vi "DblMonoPMDCurrentScanSM correction.vi"() -> ()   [LabVIEW 2010]
uses:
  <vilib>/DAQmx/write.llb/DAQmx Write (Analog DBL 1Chan 1Samp).vi
  <vilib>/DAQmx/read.llb/DAQmx Read (Analog 1D DBL 1Chan NSamp).vi
  <vilib>/DAQmx/read.llb/DAQmx Read (Analog 1D DBL NChan 1Samp).vi
  <vilib>/DAQmx/write.llb/DAQmx Write (Analog 2D DBL NChan NSamp).vi
  <vilib>/DAQmx/create/channels.llb/DAQmx Create Channel (AO-Voltage-Basic).vi
  <vilib>/DAQmx/create/channels.llb/DAQmx Create Channel (AI-Voltage-Basic).vi
  <vilib>/daqmx/miscellaneous.llb/DAQmx Fill In Error Info.vi
  <vilib>/DAQmx/configure/timing.llb/DAQmx Timing (Sample Clock).vi
  <vilib>/Utility/file.llb/Write To Spreadsheet File (DBL).vi
  <vilib>/Analysis/NI_AALBase.lvlib
panel:
  out "element 2":dbl=-0.008255603353784051
  out "element":dbl=0.0008638386633684422
  out "number of samples written per channel":u32=999
  out "Waveform Chart  Y":dbl[](graph)=[-0.007933120791494438, -0.007933631209985054, -0.007934141628475668, -0.007934652046966284, -0.0079351624654569, -0.007935672883947514, -0.00793618330243813, -0.007936693720928744, -0.00793720413941936, -0.007937714557909975, -0.00793822497640059, -0.007938735394891205, -0.007939245813381821, -0.007939756231872435, -0.007940266650363051, -0.007940777068853667, -0.007941287487344281, -0.007941797905834897, -0.007942308324325511, -0.007942818742816127, -0.007943329161306743, -0.007943839579797357, -0.007944349998287973, -0.007944860416778589, -0.007945370835269203, -0.007945881253759819, -0.007946391672250435, -0.007946902090741049, -0.007947412509231665, -0.00794792292772228, -0.007948433346212895, -0.00794894376470351, -0.007949454183194125, -0.00794996460168474, -0.007950475020175356, -0.00795098543866597, -0.007951495857156586, -0.007952006275647202, -0.007952516694137816, -0.007953027112628432, -0.007953537531119048, -0.007954047949609662, -0.007954558368100278, -0.007955068786590892, -0.007955579205081508, -0.007956089623572124, -0.007956600042062738, -0.007957110460553354, -0.00795762087904397, -0.007958131297534584, -0.0079586417160252, -0.007959152134515816, -0.00795966255300643, -0.007960172971497046, -0.00796068338998766, -0.007961193808478276, -0.007961704226968892, -0.007962214645459506, -0.007962725063950122, -0.007963235482440737, -0.007963745900931352, -0.007964256319421967, -0.007964766737912583, -0.007965277156403197, -0.007965787574893813, -0.007966297993384427, -0.007966808411875043, -0.00796731883036566, -0.007967829248856273, -0.00796833966734689, -0.007968850085837505, -0.00796936050432812, -0.007969870922818735, -0.007970381341309351, -0.007970891759799965, -0.007971402178290581, -0.007971912596781195, -0.007972423015271811, -0.007972933433762427, -0.007973443852253041, -0.007973954270743657, -0.007974464689234273, -0.007974975107724887, -0.007975485526215503, -0.007975995944706119, -0.007976506363196733, -0.007977016781687348, -0.007977527200177963, -0.007978037618668578, -0.007978548037159194, -0.007979058455649808, -0.007979568874140424, -0.00798007929263104, -0.007980589711121654, -0.00798110012961227, -0.007981610548102886, -0.0079821209665935, -0.007982631385084116, -0.007983141803574732, -0.007983652222065346, -0.007984162640555962, -0.007984673059046576, -0.007985183477537192, -0.007985693896027808, -0.007986204314518422, -0.007986714733009038, -0.007987225151499654, -0.007987735569990268, -0.007988245988480884, -0.0079887564069715, -0.007989266825462114, -0.00798977724395273, -0.007990287662443344, -0.00799079808093396, -0.007991308499424575, -0.00799181891791519, -0.007992329336405805, -0.007992839754896421, -0.007993350173387035, -0.007993860591877651, -0.007994371010368267, -0.007994881428858881, -0.007995391847349497, -0.007995902265840111, -0.007996412684330727, -0.007996923102821343, -0.007997433521311957, -0.007997943939802573, -0.007998454358293189, -0.007998964776783803, -0.007999475195274419, -0.007999985613765035, -0.008000496032255649, -0.008001006450746265, -0.00800151686923688, -0.008002027287727495, -0.00800253770621811, -0.008003048124708725, -0.00800355854319934, -0.008004068961689956, -0.00800457938018057, -0.008005089798671186, -0.008005600217161802, -0.008006110635652416, -0.008006621054143032, -0.008007131472633648, -0.008007641891124262, -0.008008152309614878, -0.008008662728105492, -0.008009173146596108, -0.008009683565086724, -0.008010193983577338, -0.008010704402067954, -0.00801121482055857, -0.008011725239049184, -0.0080122356575398, -0.008012746076030416, -0.00801325649452103, -0.008013766913011646, -0.00801427733150226, -0.008014787749992876, -0.008015298168483492, -0.008015808586974106, -0.008016319005464722, -0.008016829423955337, -0.008017339842445952, -0.008017850260936567, -0.008018360679427183, -0.008018871097917797, -0.008019381516408413, -0.008019891934899027, -0.008020402353389643, -0.00802091277188026, -0.008021423190370873, -0.00802193360886149, -0.008022444027352105, -0.00802295444584272, -0.008023464864333335, -0.008023975282823951, -0.008024485701314565, -0.008024996119805181, -0.008025506538295795, -0.008026016956786411, -0.008026527375277027, -0.008027037793767641, -0.008027548212258257, -0.008028058630748873, -0.008028569049239487, -0.008029079467730103, -0.008029589886220719, -0.008030100304711333, -0.008030610723201949, -0.008031121141692563, -0.008031631560183179, -0.008032141978673794, -0.008032652397164409, -0.008033162815655024, -0.00803367323414564, -0.008034183652636254, -0.00803469407112687, -0.008035204489617486, -0.0080357149081081, -0.008036225326598716, -0.008036735745089332, -0.008037246163579946, -0.008037756582070562, -0.008038267000561176, -0.008038777419051792, -0.008039287837542408, -0.008039798256033022, -0.008040308674523638, -0.008040819093014254, -0.008041329511504868, -0.008041839929995484, -0.0080423503484861, -0.008042860766976714, -0.00804337118546733, -0.008043881603957944, -0.00804439202244856, -0.008044902440939175, -0.00804541285942979, -0.008045923277920405, -0.008046433696411021, -0.008046944114901635, -0.008047454533392251, -0.008047964951882867, -0.008048475370373481, -0.008048985788864097, -0.008049496207354711, -0.008050006625845327, -0.008050517044335943, -0.008051027462826557, -0.008051537881317173, -0.008052048299807789, -0.008052558718298403, -0.008053069136789019, -0.008053579555279635, -0.008054089973770249, -0.008054600392260865, -0.00805511081075148, -0.008055621229242095, -0.00805613164773271, -0.008056642066223325, -0.00805715248471394, -0.008057662903204556, -0.00805817332169517, -0.008058683740185786, -0.008059194158676402, -0.008059704577167016, -0.008060214995657632, -0.008060725414148248, -0.008061235832638862, -0.008061746251129478, -0.008062256669620092, -0.008062767088110708, -0.008063277506601324, -0.008063787925091938, -0.008064298343582554, -0.00806480876207317, -0.008065319180563784, -0.0080658295990544, -0.008066340017545016, -0.00806685043603563, -0.008067360854526246, -0.00806787127301686, -0.008068381691507476, -0.008068892109998092, -0.008069402528488706, -0.008069912946979322, -0.008070423365469937, -0.008070933783960552, -0.008071444202451167, -0.008071954620941783, -0.008072465039432397, -0.008072975457923013, -0.008073485876413627, -0.008073996294904243, -0.00807450671339486, -0.008075017131885473, -0.00807552755037609, -0.008076037968866705, -0.00807654838735732, -0.008077058805847935, -0.008077569224338551, -0.008078079642829165, -0.008078590061319781, -0.008079100479810395, -0.008079610898301011, -0.008080121316791627, -0.008080631735282241, -0.008081142153772857, -0.008081652572263473, -0.008082162990754087, -0.008082673409244703, -0.008083183827735319, -0.008083694246225933, -0.008084204664716549, -0.008084715083207164, -0.008085225501697779, -0.008085735920188394, -0.008086246338679009, -0.008086756757169624, -0.00808726717566024, -0.008087777594150854, -0.00808828801264147, -0.008088798431132086, -0.0080893088496227, -0.008089819268113316, -0.008090329686603932, -0.008090840105094546, -0.008091350523585162, -0.008091860942075776, -0.008092371360566392, -0.008092881779057008, -0.008093392197547622, -0.008093902616038238, -0.008094413034528854, -0.008094923453019468, -0.008095433871510084, -0.0080959442900007, -0.008096454708491314, -0.00809696512698193, -0.008097475545472544, -0.00809798596396316, -0.008098496382453775, -0.00809900680094439, -0.008099517219435005, -0.008100027637925621, -0.008100538056416235, -0.008101048474906851, -0.008101558893397467, -0.008102069311888081, -0.008102579730378697, -0.008103090148869311, -0.008103600567359927, -0.008104110985850543, -0.008104621404341157, -0.008105131822831773, -0.008105642241322389, -0.008106152659813003, -0.008106663078303619, -0.008107173496794235, -0.008107683915284849, -0.008108194333775465, -0.008108704752266079, -0.008109215170756695, -0.00810972558924731, -0.008110236007737925, -0.00811074642622854, -0.008111256844719156, -0.00811176726320977, -0.008112277681700386, -0.008112788100191002, -0.008113298518681616, -0.008113808937172232, -0.008114319355662848, -0.008114829774153462, -0.008115340192644078, -0.008115850611134692, -0.008116361029625308, -0.008116871448115924, -0.008117381866606538, -0.008117892285097154, -0.00811840270358777, -0.008118913122078384, -0.008119423540569, -0.008119933959059616, -0.00812044437755023, -0.008120954796040846, -0.00812146521453146, -0.008121975633022076, -0.008122486051512692, -0.008122996470003306, -0.008123506888493922, -0.008124017306984537, -0.008124527725475152, -0.008125038143965767, -0.008125548562456383, -0.008126058980946997, -0.008126569399437613, -0.008127079817928227, -0.008127590236418843, -0.00812810065490946, -0.008128611073400073, -0.00812912149189069, -0.008129631910381305, -0.00813014232887192, -0.008130652747362535, -0.008131163165853151, -0.008131673584343765, -0.008132184002834381, -0.008132694421324995, -0.008133204839815611, -0.008133715258306227, -0.008134225676796841, -0.008134736095287457, -0.008135246513778073, -0.008135756932268687, -0.008136267350759303, -0.008136777769249919, -0.008137288187740533, -0.008137798606231149, -0.008138309024721764, -0.008138819443212379, -0.008139329861702994, -0.008139840280193609, -0.008140350698684224, -0.00814086111717484, -0.008141371535665454, -0.00814188195415607, -0.008142392372646686, -0.0081429027911373, -0.008143413209627916, -0.008143923628118532, -0.008144434046609146, -0.008144944465099762, -0.008145454883590376, -0.008145965302080992, -0.008146475720571608, -0.008146986139062222, -0.008147496557552838, -0.008148006976043454, -0.008148517394534068, -0.008149027813024684, -0.0081495382315153, -0.008150048650005914, -0.00815055906849653, -0.008151069486987144, -0.00815157990547776, -0.008152090323968375, -0.00815260074245899, -0.008153111160949605, -0.008153621579440221, -0.008154131997930835, -0.008154642416421451, -0.008155152834912067, -0.008155663253402681, -0.008156173671893297, -0.008156684090383911, -0.008157194508874527, -0.008157704927365143, -0.008158215345855757, -0.008158725764346373, -0.008159236182836989, -0.008159746601327603, -0.008160257019818219, -0.008160767438308835, -0.008161277856799449, -0.008161788275290065, -0.008162298693780679, -0.008162809112271295, -0.00816331953076191, -0.008163829949252525, -0.00816434036774314, -0.008164850786233756, -0.00816536120472437, -0.008165871623214986, -0.008166382041705602, -0.008166892460196216, -0.008167402878686832, -0.008167913297177448, -0.008168423715668062, -0.008168934134158678, -0.008169444552649292, -0.008169954971139908, -0.008170465389630524, -0.008170975808121138, -0.008171486226611754, -0.00817199664510237, -0.008172507063592984, -0.0081730174820836, -0.008173527900574216, -0.00817403831906483, -0.008174548737555446, -0.00817505915604606, -0.008175569574536676, -0.008176079993027292, -0.008176590411517906, -0.008177100830008522, -0.008177611248499137, -0.008178121666989752, -0.008178632085480367, -0.008179142503970983, -0.008179652922461597, -0.008180163340952213, -0.008180673759442827, -0.008181184177933443, -0.00818169459642406, -0.008182205014914673, -0.00818271543340529, -0.008183225851895905, -0.00818373627038652, -0.008184246688877135, -0.008184757107367751, -0.008185267525858365, -0.008185777944348981, -0.008186288362839595, -0.008186798781330211, -0.008187309199820827, -0.008187819618311441, -0.008188330036802057, -0.008188840455292673, -0.008189350873783287, -0.008189861292273903, -0.008190371710764519, -0.008190882129255133, -0.008191392547745749, -0.008191902966236363, -0.008192413384726979, -0.008192923803217594, -0.008193434221708209, -0.008193944640198824, -0.00819445505868944, -0.008194965477180054, -0.00819547589567067, -0.008195986314161286, -0.0081964967326519, -0.008197007151142516, -0.00819751756963313, -0.008198027988123746, -0.008198538406614362, -0.008199048825104976, -0.008199559243595592, -0.008200069662086208, -0.008200580080576822, -0.008201090499067438, -0.008201600917558054, -0.008202111336048668, -0.008202621754539284, -0.008203132173029898, -0.008203642591520514, -0.00820415301001113, -0.008204663428501744, -0.00820517384699236, -0.008205684265482975, -0.00820619468397359, -0.008206705102464205, -0.008207215520954821, -0.008207725939445435, -0.008208236357936051, -0.008208746776426667, -0.008209257194917281, -0.008209767613407897, -0.008210278031898511, -0.008210788450389127, -0.008211298868879743, -0.008211809287370357, -0.008212319705860973, -0.008212830124351589, -0.008213340542842203, -0.008213850961332819, -0.008214361379823435, -0.008214871798314049, -0.008215382216804665, -0.008215892635295279, -0.008216403053785895, -0.00821691347227651, -0.008217423890767125, -0.00821793430925774, -0.008218444727748356, -0.00821895514623897, -0.008219465564729586, -0.008219975983220202, -0.008220486401710816, -0.008220996820201432, -0.008221507238692046, -0.008222017657182662, -0.008222528075673278, -0.008223038494163892, -0.008223548912654508, -0.008224059331145124, -0.008224569749635738, -0.008225080168126354, -0.00822559058661697, -0.008226101005107584, -0.0082266114235982, -0.008227121842088816, -0.00822763226057943, -0.008228142679070046, -0.00822865309756066, -0.008229163516051276, -0.008229673934541892, -0.008230184353032506, -0.008230694771523122, -0.008231205190013738, -0.008231715608504352, -0.008232226026994967, -0.008232736445485583, -0.008233246863976197, -0.008233757282466813, -0.008234267700957427, -0.008234778119448043, -0.00823528853793866, -0.008235798956429273, -0.00823630937491989, -0.008236819793410505, -0.00823733021190112, -0.008237840630391735, -0.008238351048882351, -0.008238861467372965, -0.008239371885863581, -0.008239882304354195, -0.008240392722844811, -0.008240903141335427, -0.008241413559826041, -0.008241923978316657, -0.008242434396807273, -0.008242944815297887, -0.008243455233788503, -0.008243965652279119, -0.008244476070769733, -0.008244986489260349, -0.008245496907750963, -0.008246007326241579, -0.008246517744732194, -0.008247028163222809, -0.008247538581713424, -0.00824804900020404, -0.008248559418694654, -0.00824906983718527, -0.008249580255675886, -0.0082500906741665, -0.008250601092657116, -0.00825111151114773, -0.008251621929638346, -0.008252132348128962, -0.008252642766619576, -0.008253153185110192, -0.008253663603600808, -0.008254174022091422, -0.008254684440582038, -0.008255194859072654, -0.008255705277563268, -0.008256215696053884, -0.008256726114544498, -0.008257236533035114, -0.00825774695152573, -0.008258257370016344, -0.00825876778850696, -0.008259278206997575, -0.00825978862548819, -0.008260299043978805, -0.008260809462469421, -0.008261319880960035, -0.008261830299450651, -0.008262340717941265, -0.008262851136431881, -0.008263361554922497, -0.008263871973413111, -0.008264382391903727, -0.008264892810394343, -0.008265403228884957, -0.008265913647375573, -0.008266424065866189, -0.008266934484356803, -0.008267444902847419, -0.008267955321338035, -0.008268465739828649, -0.008268976158319265, -0.008269486576809879, -0.008269996995300495, -0.00827050741379111, -0.008271017832281725, -0.00827152825077234, -0.008272038669262956, -0.00827254908775357, -0.008273059506244186, -0.008273569924734802, -0.008274080343225416, -0.008274590761716032, -0.008275101180206646, -0.008275611598697262, -0.008276122017187878, -0.008276632435678492, -0.008277142854169108, -0.008277653272659724, -0.008278163691150338, -0.008278674109640954, -0.00827918452813157, -0.008279694946622184, -0.0082802053651128, -0.008280715783603416, -0.00828122620209403, -0.008281736620584646, -0.00828224703907526, -0.008282757457565876, -0.008283267876056492, -0.008283778294547106, -0.008284288713037722, -0.008284799131528338, -0.008285309550018952, -0.008285819968509568, -0.008286330387000183, -0.008286840805490798, -0.008287351223981413, -0.008287861642472028, -0.008288372060962643, -0.00828888247945326, -0.008289392897943873, -0.00828990331643449, -0.008290413734925105, -0.00829092415341572, -0.008291434571906335, -0.008291944990396951, -0.008292455408887565, -0.008292965827378181, -0.008293476245868795, -0.008293986664359411, -0.008294497082850027, -0.008295007501340641, -0.008295517919831257, -0.008296028338321873, -0.008296538756812487, -0.008297049175303103, -0.008297559593793719, -0.008298070012284333, -0.008298580430774949, -0.008299090849265563, -0.008299601267756179, -0.008300111686246794, -0.008300622104737409, -0.008301132523228024, -0.00830164294171864, -0.008302153360209254, -0.00830266377869987, -0.008303174197190486, -0.0083036846156811, -0.008304195034171716, -0.00830470545266233, -0.008305215871152946, -0.008305726289643562, -0.008306236708134176, -0.008306747126624792, -0.008307257545115408, -0.008307767963606022, -0.008308278382096638, -0.008308788800587254, -0.008309299219077868, -0.008309809637568484, -0.008310320056059098, -0.008310830474549714, -0.00831134089304033, -0.008311851311530944, -0.00831236173002156, -0.008312872148512175, -0.00831338256700279, -0.008313892985493405, -0.008314403403984021, -0.008314913822474635, -0.008315424240965251, -0.008315934659455865, -0.008316445077946481, -0.008316955496437097, -0.008317465914927711, -0.008317976333418327, -0.008318486751908943, -0.008318997170399557, -0.008319507588890173, -0.008320018007380789, -0.008320528425871403, -0.008321038844362019, -0.008321549262852633, -0.008322059681343249, -0.008322570099833865, -0.008323080518324479, -0.008323590936815095, -0.00832410135530571, -0.008324611773796325, -0.00832512219228694, -0.008325632610777556, -0.00832614302926817, -0.008326653447758786, -0.008327163866249402, -0.008327674284740016, -0.008328184703230632, -0.008328695121721246, -0.008329205540211862, -0.008329715958702478, -0.008330226377193092, -0.008330736795683708, -0.008331247214174324, -0.008331757632664938, -0.008332268051155554, -0.00833277846964617, -0.008333288888136784, -0.0083337993066274, -0.008334309725118014, -0.00833482014360863, -0.008335330562099246, -0.00833584098058986, -0.008336351399080476, -0.008336861817571092, -0.008337372236061706, -0.008337882654552322, -0.008338393073042938, -0.008338903491533552, -0.008339413910024168, -0.008339924328514783, -0.008340434747005398, -0.008340945165496013, -0.008341455583986628, -0.008341966002477243, -0.00834247642096786, -0.008342986839458473, -0.00834349725794909, -0.008344007676439705, -0.00834451809493032, -0.008345028513420935, -0.008345538931911551, -0.008346049350402165, -0.008346559768892781, -0.008347070187383395, -0.008347580605874011, -0.008348091024364627, -0.008348601442855241, -0.008349111861345857, -0.008349622279836473, -0.008350132698327087, -0.008350643116817703, -0.008351153535308319, -0.008351663953798933, -0.008352174372289549, -0.008352684790780163, -0.008353195209270779, -0.008353705627761394, -0.008354216046252009, -0.008354726464742624, -0.00835523688323324, -0.008355747301723854, -0.00835625772021447, -0.008356768138705086, -0.0083572785571957, -0.008357788975686316, -0.00835829939417693, -0.008358809812667546, -0.008359320231158162, -0.008359830649648776, -0.008360341068139392, -0.008360851486630008, -0.008361361905120622, -0.008361872323611238, -0.008362382742101854, -0.008362893160592468, -0.008363403579083084, -0.008363913997573698, -0.008364424416064314, -0.00836493483455493, -0.008365445253045544, -0.00836595567153616, -0.008366466090026775, -0.00836697650851739, -0.008367486927008005, -0.008367997345498621, -0.008368507763989235, -0.008369018182479851, -0.008369528600970465, -0.008370039019461081, -0.008370549437951697, -0.008371059856442311, -0.008371570274932927, -0.008372080693423543, -0.008372591111914157, -0.008373101530404773, -0.008373611948895389, -0.008374122367386003, -0.008374632785876619, -0.008375143204367233, -0.008375653622857849, -0.008376164041348465, -0.008376674459839079, -0.008377184878329695, -0.00837769529682031, -0.008378205715310925, -0.00837871613380154, -0.008379226552292156, -0.00837973697078277, -0.008380247389273386, -0.008380757807764002, -0.008381268226254616, -0.008381778644745232, -0.008382289063235846, -0.008382799481726462, -0.008383309900217078, -0.008383820318707692, -0.008384330737198308, -0.008384841155688924, -0.008385351574179538, -0.008385861992670154, -0.00838637241116077, -0.008386882829651384, -0.008387393248142, -0.008387903666632614, -0.00838841408512323, -0.008388924503613846, -0.00838943492210446, -0.008389945340595076, -0.008390455759085692, -0.008390966177576306, -0.008391476596066922, -0.008391987014557538, -0.008392497433048152, -0.008393007851538768, -0.008393518270029383, -0.008394028688519998, -0.008394539107010613, -0.008395049525501228, -0.008395559943991843, -0.00839607036248246, -0.008396580780973073, -0.00839709119946369, -0.008397601617954305, -0.00839811203644492, -0.008398622454935535, -0.008399132873426151, -0.008399643291916765, -0.008400153710407381, -0.008400664128897995, -0.008401174547388611, -0.008401684965879227, -0.008402195384369841, -0.008402705802860457, -0.008403216221351073, -0.008403726639841687, -0.008404237058332303, -0.008404747476822919, -0.008405257895313533, -0.008405768313804149, -0.008406278732294763, -0.008406789150785379, -0.008407299569275994, -0.008407809987766609, -0.008408320406257224, -0.00840883082474784, -0.008409341243238454, -0.00840985166172907, -0.008410362080219686, -0.0084108724987103, -0.008411382917200916, -0.00841189333569153, -0.008412403754182146, -0.008412914172672762, -0.008413424591163376, -0.008413935009653992, -0.008414445428144608, -0.008414955846635222, -0.008415466265125838, -0.008415976683616454, -0.008416487102107068, -0.008416997520597684, -0.008417507939088298, -0.008418018357578914, -0.00841852877606953, -0.008419039194560144, -0.00841954961305076, -0.008420060031541375, -0.00842057045003199, -0.008421080868522605, -0.008421591287013221, -0.008422101705503835, -0.008422612123994451, -0.008423122542485065, -0.008423632960975681, -0.008424143379466297, -0.008424653797956911, -0.008425164216447527, -0.008425674634938143, -0.008426185053428757, -0.008426695471919373, -0.008427205890409989, -0.008427716308900603, -0.008428226727391219, -0.008428737145881835, -0.008429247564372449, -0.008429757982863065, -0.008430268401353679, -0.008430778819844295, -0.00843128923833491, -0.008431799656825525, -0.00843231007531614, -0.008432820493806756, -0.00843333091229737, -0.008433841330787986, -0.0084343517492786, -0.008434862167769216, -0.008435372586259832, -0.008435883004750446, -0.008436393423241062, -0.008436903841731678, -0.008437414260222292, -0.008437924678712908, -0.008438435097203524, -0.008438945515694138, -0.008439455934184754, -0.00843996635267537, -0.008440476771165984, -0.0084409871896566, -0.008441497608147216, -0.00844200802663783, -0.008442518445128446, -0.00844302886361906]
  out "initial y":dbl=-0.007933120791494438
  out "Final Y":dbl=-0.00844302886361906
  out "Waveform Chart X":dbl[](graph)=[0.0015088037910843937, 0.0015086913782654677, 0.0015085789654465417, 0.0015084665526276157, 0.00150835413980869, 0.001508241726989764, 0.001508129314170838, 0.001508016901351912, 0.001507904488532986, 0.00150779207571406, 0.001507679662895134, 0.0015075672500762082, 0.0015074548372572823, 0.0015073424244383563, 0.0015072300116194303, 0.0015071175988005043, 0.0015070051859815783, 0.0015068927731626523, 0.0015067803603437265, 0.0015066679475248005, 0.0015065555347058745, 0.0015064431218869486, 0.0015063307090680226, 0.0015062182962490966, 0.0015061058834301706, 0.0015059934706112446, 0.0015058810577923188, 0.0015057686449733928, 0.0015056562321544668, 0.0015055438193355408, 0.0015054314065166149, 0.0015053189936976889, 0.0015052065808787629, 0.001505094168059837, 0.0015049817552409111, 0.0015048693424219851, 0.0015047569296030591, 0.0015046445167841331, 0.0015045321039652072, 0.0015044196911462812, 0.0015043072783273554, 0.0015041948655084294, 0.0015040824526895034, 0.0015039700398705774, 0.0015038576270516514, 0.0015037452142327254, 0.0015036328014137994, 0.0015035203885948737, 0.0015034079757759477, 0.0015032955629570217, 0.0015031831501380957, 0.0015030707373191697, 0.0015029583245002437, 0.0015028459116813177, 0.001502733498862392, 0.001502621086043466, 0.00150250867322454, 0.001502396260405614, 0.001502283847586688, 0.001502171434767762, 0.001502059021948836, 0.0015019466091299102, 0.0015018341963109842, 0.0015017217834920583, 0.0015016093706731323, 0.0015014969578542063, 0.0015013845450352803, 0.0015012721322163543, 0.0015011597193974285, 0.0015010473065785025, 0.0015009348937595765, 0.0015008224809406505, 0.0015007100681217246, 0.0015005976553027986, 0.0015004852424838726, 0.0015003728296649468, 0.0015002604168460208, 0.0015001480040270948, 0.0015000355912081688, 0.0014999231783892428, 0.0014998107655703169, 0.0014996983527513909, 0.0014995859399324649, 0.001499473527113539, 0.001499361114294613, 0.0014992487014756871, 0.0014991362886567611, 0.0014990238758378351, 0.0014989114630189091, 0.0014987990501999832, 0.0014986866373810574, 0.0014985742245621314, 0.0014984618117432054, 0.0014983493989242794, 0.0014982369861053534, 0.0014981245732864274, 0.0014980121604675014, 0.0014978997476485757, 0.0014977873348296497, 0.0014976749220107237, 0.0014975625091917977, 0.0014974500963728717, 0.0014973376835539457, 0.0014972252707350197, 0.001497112857916094, 0.001497000445097168, 0.001496888032278242, 0.001496775619459316, 0.00149666320664039, 0.001496550793821464, 0.001496438381002538, 0.0014963259681836122, 0.0014962135553646862, 0.0014961011425457602, 0.0014959887297268343, 0.0014958763169079083, 0.0014957639040889823, 0.0014956514912700563, 0.0014955390784511305, 0.0014954266656322045, 0.0014953142528132785, 0.0014952018399943525, 0.0014950894271754266, 0.0014949770143565006, 0.0014948646015375746, 0.0014947521887186486, 0.0014946397758997228, 0.0014945273630807968, 0.0014944149502618708, 0.0014943025374429448, 0.0014941901246240188, 0.0014940777118050929, 0.0014939652989861669, 0.001493852886167241, 0.001493740473348315, 0.0014936280605293891, 0.0014935156477104631, 0.0014934032348915371, 0.0014932908220726111, 0.0014931784092536851, 0.0014930659964347594, 0.0014929535836158334, 0.0014928411707969074, 0.0014927287579779814, 0.0014926163451590554, 0.0014925039323401294, 0.0014923915195212034, 0.0014922791067022777, 0.0014921666938833517, 0.0014920542810644257, 0.0014919418682454997, 0.0014918294554265737, 0.0014917170426076477, 0.0014916046297887217, 0.001491492216969796, 0.00149137980415087, 0.001491267391331944, 0.001491154978513018, 0.001491042565694092, 0.001490930152875166, 0.00149081774005624, 0.0014907053272373142, 0.0014905929144183882, 0.0014904805015994622, 0.0014903680887805363, 0.0014902556759616103, 0.0014901432631426843, 0.0014900308503237583, 0.0014899184375048325, 0.0014898060246859065, 0.0014896936118669805, 0.0014895811990480545, 0.0014894687862291285, 0.0014893563734102026, 0.0014892439605912766, 0.0014891315477723508, 0.0014890191349534248, 0.0014889067221344988, 0.0014887943093155728, 0.0014886818964966468, 0.0014885694836777208, 0.0014884570708587948, 0.0014883446580398689, 0.001488232245220943, 0.001488119832402017, 0.001488007419583091, 0.0014878950067641651, 0.0014877825939452391, 0.0014876701811263131, 0.0014875577683073871, 0.0014874453554884614, 0.0014873329426695354, 0.0014872205298506094, 0.0014871081170316834, 0.0014869957042127574, 0.0014868832913938314, 0.0014867708785749054, 0.0014866584657559797, 0.0014865460529370537, 0.0014864336401181277, 0.0014863212272992017, 0.0014862088144802757, 0.0014860964016613497, 0.0014859839888424237, 0.001485871576023498, 0.001485759163204572, 0.001485646750385646, 0.00148553433756672, 0.001485421924747794, 0.001485309511928868, 0.001485197099109942, 0.001485084686291016, 0.0014849722734720902, 0.0014848598606531642, 0.0014847474478342382, 0.0014846350350153123, 0.0014845226221963863, 0.0014844102093774603, 0.0014842977965585343, 0.0014841853837396085, 0.0014840729709206825, 0.0014839605581017565, 0.0014838481452828305, 0.0014837357324639045, 0.0014836233196449786, 0.0014835109068260526, 0.0014833984940071268, 0.0014832860811882008, 0.0014831736683692748, 0.0014830612555503488, 0.0014829488427314228, 0.0014828364299124968, 0.0014827240170935709, 0.001482611604274645, 0.001482499191455719, 0.001482386778636793, 0.001482274365817867, 0.0014821619529989411, 0.0014820495401800151, 0.0014819371273610891, 0.0014818247145421634, 0.0014817123017232374, 0.0014815998889043114, 0.0014814874760853854, 0.0014813750632664594, 0.0014812626504475334, 0.0014811502376286074, 0.0014810378248096816, 0.0014809254119907557, 0.0014808129991718297, 0.0014807005863529037, 0.0014805881735339777, 0.0014804757607150517, 0.0014803633478961257, 0.0014802509350772, 0.001480138522258274, 0.001480026109439348, 0.001479913696620422, 0.001479801283801496, 0.00147968887098257, 0.001479576458163644, 0.0014794640453447182, 0.0014793516325257922, 0.0014792392197068662, 0.0014791268068879402, 0.0014790143940690142, 0.0014789019812500883, 0.0014787895684311623, 0.0014786771556122363, 0.0014785647427933105, 0.0014784523299743845, 0.0014783399171554585, 0.0014782275043365325, 0.0014781150915176065, 0.0014780026786986806, 0.0014778902658797546, 0.0014777778530608288, 0.0014776654402419028, 0.0014775530274229768, 0.0014774406146040508, 0.0014773282017851248, 0.0014772157889661988, 0.0014771033761472728, 0.001476990963328347, 0.001476878550509421, 0.001476766137690495, 0.001476653724871569, 0.0014765413120526431, 0.0014764288992337171, 0.0014763164864147911, 0.0014762040735958654, 0.0014760916607769394, 0.0014759792479580134, 0.0014758668351390874, 0.0014757544223201614, 0.0014756420095012354, 0.0014755295966823094, 0.0014754171838633836, 0.0014753047710444576, 0.0014751923582255317, 0.0014750799454066057, 0.0014749675325876797, 0.0014748551197687537, 0.0014747427069498277, 0.001474630294130902, 0.001474517881311976, 0.00147440546849305, 0.001474293055674124, 0.001474180642855198, 0.001474068230036272, 0.001473955817217346, 0.0014738434043984202, 0.0014737309915794942, 0.0014736185787605682, 0.0014735061659416422, 0.0014733937531227162, 0.0014732813403037903, 0.0014731689274848643, 0.0014730565146659383, 0.0014729441018470125, 0.0014728316890280865, 0.0014727192762091605, 0.0014726068633902345, 0.0014724944505713085, 0.0014723820377523825, 0.0014722696249334566, 0.0014721572121145308, 0.0014720447992956048, 0.0014719323864766788, 0.0014718199736577528, 0.0014717075608388268, 0.0014715951480199008, 0.0014714827352009748, 0.001471370322382049, 0.001471257909563123, 0.001471145496744197, 0.001471033083925271, 0.001470920671106345, 0.0014708082582874191, 0.0014706958454684931, 0.0014705834326495673, 0.0014704710198306414, 0.0014703586070117154, 0.0014702461941927894, 0.0014701337813738634, 0.0014700213685549374, 0.0014699089557360114, 0.0014697965429170856, 0.0014696841300981596, 0.0014695717172792336, 0.0014694593044603077, 0.0014693468916413817, 0.0014692344788224557, 0.0014691220660035297, 0.001469009653184604, 0.001468897240365678, 0.001468784827546752, 0.001468672414727826, 0.0014685600019089, 0.001468447589089974, 0.001468335176271048, 0.0014682227634521222, 0.0014681103506331962, 0.0014679979378142702, 0.0014678855249953442, 0.0014677731121764182, 0.0014676606993574922, 0.0014675482865385663, 0.0014674358737196403, 0.0014673234609007145, 0.0014672110480817885, 0.0014670986352628625, 0.0014669862224439365, 0.0014668738096250105, 0.0014667613968060845, 0.0014666489839871585, 0.0014665365711682328, 0.0014664241583493068, 0.0014663117455303808, 0.0014661993327114548, 0.0014660869198925288, 0.0014659745070736028, 0.0014658620942546768, 0.001465749681435751, 0.001465637268616825, 0.001465524855797899, 0.001465412442978973, 0.001465300030160047, 0.001465187617341121, 0.0014650752045221951, 0.0014649627917032693, 0.0014648503788843434, 0.0014647379660654174, 0.0014646255532464914, 0.0014645131404275654, 0.0014644007276086394, 0.0014642883147897134, 0.0014641759019707876, 0.0014640634891518616, 0.0014639510763329356, 0.0014638386635140097, 0.0014637262506950837, 0.0014636138378761577, 0.0014635014250572317, 0.001463389012238306, 0.00146327659941938, 0.001463164186600454, 0.001463051773781528, 0.001462939360962602, 0.001462826948143676, 0.00146271453532475, 0.0014626021225058242, 0.0014624897096868982, 0.0014623772968679722, 0.0014622648840490462, 0.0014621524712301202, 0.0014620400584111942, 0.0014619276455922682, 0.0014618152327733423, 0.0014617028199544165, 0.0014615904071354905, 0.0014614779943165645, 0.0014613655814976385, 0.0014612531686787125, 0.0014611407558597865, 0.0014610283430408605, 0.0014609159302219348, 0.0014608035174030088, 0.0014606911045840828, 0.0014605786917651568, 0.0014604662789462308, 0.0014603538661273048, 0.0014602414533083788, 0.001460129040489453, 0.001460016627670527, 0.001459904214851601, 0.001459791802032675, 0.001459679389213749, 0.001459566976394823, 0.001459454563575897, 0.0014593421507569713, 0.0014592297379380453, 0.0014591173251191194, 0.0014590049123001934, 0.0014588924994812674, 0.0014587800866623414, 0.0014586676738434154, 0.0014585552610244896, 0.0014584428482055636, 0.0014583304353866376, 0.0014582180225677116, 0.0014581056097487857, 0.0014579931969298597, 0.0014578807841109337, 0.001457768371292008, 0.001457655958473082, 0.001457543545654156, 0.00145743113283523, 0.001457318720016304, 0.001457206307197378, 0.001457093894378452, 0.0014569814815595262, 0.0014568690687406002, 0.0014567566559216742, 0.0014566442431027482, 0.0014565318302838222, 0.0014564194174648962, 0.0014563070046459702, 0.0014561945918270443, 0.0014560821790081185, 0.0014559697661891925, 0.0014558573533702665, 0.0014557449405513405, 0.0014556325277324145, 0.0014555201149134885, 0.0014554077020945625, 0.0014552952892756368, 0.0014551828764567108, 0.0014550704636377848, 0.0014549580508188588, 0.0014548456379999328, 0.0014547332251810068, 0.0014546208123620808, 0.001454508399543155, 0.001454395986724229, 0.001454283573905303, 0.001454171161086377, 0.001454058748267451, 0.001453946335448525, 0.001453833922629599, 0.0014537215098106733, 0.0014536090969917473, 0.0014534966841728213, 0.0014533842713538954, 0.0014532718585349694, 0.0014531594457160434, 0.0014530470328971174, 0.0014529346200781916, 0.0014528222072592656, 0.0014527097944403396, 0.0014525973816214136, 0.0014524849688024876, 0.0014523725559835617, 0.0014522601431646357, 0.00145214773034571, 0.001452035317526784, 0.001451922904707858, 0.001451810491888932, 0.001451698079070006, 0.00145158566625108, 0.001451473253432154, 0.0014513608406132282, 0.0014512484277943022, 0.0014511360149753762, 0.0014510236021564502, 0.0014509111893375242, 0.0014507987765185982, 0.0014506863636996722, 0.0014505739508807462, 0.0014504615380618205, 0.0014503491252428945, 0.0014502367124239685, 0.0014501242996050425, 0.0014500118867861165, 0.0014498994739671905, 0.0014497870611482645, 0.0014496746483293388, 0.0014495622355104128, 0.0014494498226914868, 0.0014493374098725608, 0.0014492249970536348, 0.0014491125842347088, 0.001449000171415783, 0.001448887758596857, 0.001448775345777931, 0.001448662932959005, 0.001448550520140079, 0.001448438107321153, 0.001448325694502227, 0.001448213281683301, 0.0014481008688643753, 0.0014479884560454493, 0.0014478760432265233, 0.0014477636304075973, 0.0014476512175886714, 0.0014475388047697454, 0.0014474263919508194, 0.0014473139791318936, 0.0014472015663129676, 0.0014470891534940416, 0.0014469767406751156, 0.0014468643278561896, 0.0014467519150372637, 0.0014466395022183377, 0.0014465270893994119, 0.001446414676580486, 0.00144630226376156, 0.001446189850942634, 0.001446077438123708, 0.001445965025304782, 0.001445852612485856, 0.0014457401996669302, 0.0014456277868480042, 0.0014455153740290782, 0.0014454029612101522, 0.0014452905483912262, 0.0014451781355723002, 0.0014450657227533742, 0.0014449533099344482, 0.0014448408971155225, 0.0014447284842965965, 0.0014446160714776705, 0.0014445036586587445, 0.0014443912458398185, 0.0014442788330208925, 0.0014441664202019667, 0.0014440540073830407, 0.0014439415945641148, 0.0014438291817451888, 0.0014437167689262628, 0.0014436043561073368, 0.0014434919432884108, 0.001443379530469485, 0.001443267117650559, 0.001443154704831633, 0.001443042292012707, 0.001442929879193781, 0.001442817466374855, 0.001442705053555929, 0.001442592640737003, 0.0014424802279180773, 0.0014423678150991513, 0.0014422554022802253, 0.0014421429894612993, 0.0014420305766423734, 0.0014419181638234474, 0.0014418057510045214, 0.0014416933381855956, 0.0014415809253666696, 0.0014414685125477436, 0.0014413560997288176, 0.0014412436869098916, 0.0014411312740909656, 0.0014410188612720397, 0.0014409064484531139, 0.0014407940356341879, 0.001440681622815262, 0.001440569209996336, 0.00144045679717741, 0.001440344384358484, 0.001440231971539558, 0.0014401195587206322, 0.0014400071459017062, 0.0014398947330827802, 0.0014397823202638542, 0.0014396699074449282, 0.0014395574946260022, 0.0014394450818070762, 0.0014393326689881502, 0.0014392202561692245, 0.0014391078433502985, 0.0014389954305313725, 0.0014388830177124465, 0.0014387706048935205, 0.0014386581920745945, 0.0014385457792556685, 0.0014384333664367427, 0.0014383209536178168, 0.0014382085407988908, 0.0014380961279799648, 0.0014379837151610388, 0.0014378713023421128, 0.0014377588895231868, 0.001437646476704261, 0.001437534063885335, 0.001437421651066409, 0.001437309238247483, 0.001437196825428557, 0.001437084412609631, 0.001436971999790705, 0.0014368595869717793, 0.0014367471741528533, 0.0014366347613339273, 0.0014365223485150013, 0.0014364099356960753, 0.0014362975228771494, 0.0014361851100582234, 0.0014360726972392976, 0.0014359602844203716, 0.0014358478716014456, 0.0014357354587825196, 0.0014356230459635936, 0.0014355106331446676, 0.0014353982203257416, 0.0014352858075068159, 0.0014351733946878899, 0.001435060981868964, 0.001434948569050038, 0.001434836156231112, 0.001434723743412186, 0.00143461133059326, 0.0014344989177743342, 0.0014343865049554082, 0.0014342740921364822, 0.0014341616793175562, 0.0014340492664986302, 0.0014339368536797042, 0.0014338244408607782, 0.0014337120280418522, 0.0014335996152229265, 0.0014334872024040005, 0.0014333747895850745, 0.0014332623767661485, 0.0014331499639472225, 0.0014330375511282965, 0.0014329251383093707, 0.0014328127254904447, 0.0014327003126715187, 0.0014325878998525928, 0.0014324754870336668, 0.0014323630742147408, 0.0014322506613958148, 0.001432138248576889, 0.001432025835757963, 0.001431913422939037, 0.001431801010120111, 0.001431688597301185, 0.001431576184482259, 0.001431463771663333, 0.001431351358844407, 0.0014312389460254813, 0.0014311265332065553, 0.0014310141203876293, 0.0014309017075687033, 0.0014307892947497773, 0.0014306768819308513, 0.0014305644691119254, 0.0014304520562929996, 0.0014303396434740736, 0.0014302272306551476, 0.0014301148178362216, 0.0014300024050172956, 0.0014298899921983696, 0.0014297775793794436, 0.0014296651665605179, 0.0014295527537415919, 0.0014294403409226659, 0.00142932792810374, 0.001429215515284814, 0.001429103102465888, 0.001428990689646962, 0.0014288782768280362, 0.0014287658640091102, 0.0014286534511901842, 0.0014285410383712582, 0.0014284286255523322, 0.0014283162127334062, 0.0014282037999144802, 0.0014280913870955542, 0.0014279789742766284, 0.0014278665614577025, 0.0014277541486387765, 0.0014276417358198505, 0.0014275293230009245, 0.0014274169101819985, 0.0014273044973630725, 0.0014271920845441467, 0.0014270796717252207, 0.0014269672589062947, 0.0014268548460873688, 0.0014267424332684428, 0.0014266300204495168, 0.0014265176076305908, 0.001426405194811665, 0.001426292781992739, 0.001426180369173813, 0.001426067956354887, 0.001425955543535961, 0.001425843130717035, 0.001425730717898109, 0.0014256183050791833, 0.0014255058922602573, 0.0014253934794413313, 0.0014252810666224053, 0.0014251686538034793, 0.0014250562409845533, 0.0014249438281656274, 0.0014248314153467016, 0.0014247190025277756, 0.0014246065897088496, 0.0014244941768899236, 0.0014243817640709976, 0.0014242693512520716, 0.0014241569384331456, 0.0014240445256142199, 0.0014239321127952939, 0.0014238196999763679, 0.0014237072871574419, 0.001423594874338516, 0.00142348246151959, 0.001423370048700664, 0.0014232576358817381, 0.0014231452230628122, 0.0014230328102438862, 0.0014229203974249602, 0.0014228079846060342, 0.0014226955717871082, 0.0014225831589681822, 0.0014224707461492562, 0.0014223583333303304, 0.0014222459205114044, 0.0014221335076924785, 0.0014220210948735525, 0.0014219086820546265, 0.0014217962692357005, 0.0014216838564167747, 0.0014215714435978487, 0.0014214590307789227, 0.0014213466179599967, 0.0014212342051410707, 0.0014211217923221448, 0.0014210093795032188, 0.001420896966684293, 0.001420784553865367, 0.001420672141046441, 0.001420559728227515, 0.001420447315408589, 0.001420334902589663, 0.001420222489770737, 0.001420110076951811, 0.0014199976641328853, 0.0014198852513139593, 0.0014197728384950333, 0.0014196604256761073, 0.0014195480128571813, 0.0014194356000382553, 0.0014193231872193293, 0.0014192107744004036, 0.0014190983615814776, 0.0014189859487625516, 0.0014188735359436256, 0.0014187611231246996, 0.0014186487103057736, 0.0014185362974868476, 0.0014184238846679219, 0.0014183114718489959, 0.0014181990590300699, 0.0014180866462111439, 0.001417974233392218, 0.001417861820573292, 0.001417749407754366, 0.0014176369949354401, 0.0014175245821165141, 0.0014174121692975882, 0.0014172997564786622, 0.0014171873436597362, 0.0014170749308408102, 0.0014169625180218842, 0.0014168501052029582, 0.0014167376923840324, 0.0014166252795651064, 0.0014165128667461804, 0.0014164004539272545, 0.0014162880411083285, 0.0014161756282894025, 0.0014160632154704765, 0.0014159508026515507, 0.0014158383898326247, 0.0014157259770136987, 0.0014156135641947727, 0.0014155011513758468, 0.0014153887385569208, 0.0014152763257379948, 0.001415163912919069, 0.001415051500100143, 0.001414939087281217, 0.001414826674462291, 0.001414714261643365, 0.001414601848824439, 0.001414489436005513, 0.0014143770231865873, 0.0014142646103676613, 0.0014141521975487353, 0.0014140397847298093, 0.0014139273719108833, 0.0014138149590919573, 0.0014137025462730313, 0.0014135901334541056, 0.0014134777206351796, 0.0014133653078162536, 0.0014132528949973276, 0.0014131404821784016, 0.0014130280693594756, 0.0014129156565405496, 0.0014128032437216238, 0.0014126908309026979, 0.0014125784180837719, 0.0014124660052648459, 0.0014123535924459199, 0.001412241179626994, 0.001412128766808068, 0.0014120163539891421, 0.0014119039411702161, 0.0014117915283512902, 0.0014116791155323642, 0.0014115667027134382, 0.0014114542898945122, 0.0014113418770755862, 0.0014112294642566604, 0.0014111170514377344, 0.0014110046386188084, 0.0014108922257998824, 0.0014107798129809565, 0.0014106674001620305, 0.0014105549873431045, 0.0014104425745241787, 0.0014103301617052527, 0.0014102177488863267, 0.0014101053360674007, 0.0014099929232484747, 0.0014098805104295487, 0.0014097680976106228, 0.001409655684791697, 0.001409543271972771, 0.001409430859153845, 0.001409318446334919, 0.001409206033515993, 0.001409093620697067, 0.001408981207878141, 0.001408868795059215, 0.0014087563822402893, 0.0014086439694213633, 0.0014085315566024373, 0.0014084191437835113, 0.0014083067309645853, 0.0014081943181456593, 0.0014080819053267333, 0.0014079694925078076, 0.0014078570796888816, 0.0014077446668699556, 0.0014076322540510296, 0.0014075198412321036, 0.0014074074284131776, 0.0014072950155942516, 0.0014071826027753258, 0.0014070701899563999, 0.0014069577771374739, 0.0014068453643185479, 0.0014067329514996219, 0.0014066205386806959, 0.00140650812586177, 0.0014063957130428441, 0.0014062833002239181, 0.0014061708874049921, 0.0014060584745860662, 0.0014059460617671402, 0.0014058336489482142, 0.0014057212361292882, 0.0014056088233103622, 0.0014054964104914364, 0.0014053839976725104, 0.0014052715848535844, 0.0014051591720346584, 0.0014050467592157325, 0.0014049343463968065, 0.0014048219335778805, 0.0014047095207589547, 0.0014045971079400287, 0.0014044846951211027, 0.0014043722823021767, 0.0014042598694832507, 0.0014041474566643247, 0.0014040350438453988, 0.001403922631026473, 0.001403810218207547, 0.001403697805388621, 0.001403585392569695, 0.001403472979750769, 0.001403360566931843, 0.001403248154112917, 0.0014031357412939913, 0.0014030233284750653, 0.0014029109156561393, 0.0014027985028372133, 0.0014026860900182873, 0.0014025736771993613, 0.0014024612643804353, 0.0014023488515615096, 0.0014022364387425836, 0.0014021240259236576, 0.0014020116131047316, 0.0014018992002858056, 0.0014017867874668796, 0.0014016743746479536, 0.0014015619618290276, 0.0014014495490101018, 0.0014013371361911759, 0.0014012247233722499, 0.0014011123105533239, 0.0014009998977343979, 0.0014008874849154719, 0.001400775072096546, 0.0014006626592776201, 0.0014005502464586941, 0.0014004378336397681, 0.0014003254208208422, 0.0014002130080019162, 0.0014001005951829902, 0.0013999881823640644, 0.0013998757695451384, 0.0013997633567262124, 0.0013996509439072864, 0.0013995385310883604, 0.0013994261182694344, 0.0013993137054505085, 0.0013992012926315827, 0.0013990888798126567, 0.0013989764669937307, 0.0013988640541748047, 0.0013987516413558787, 0.0013986392285369527, 0.0013985268157180267, 0.001398414402899101, 0.001398301990080175, 0.001398189577261249, 0.001398077164442323, 0.001397964751623397, 0.001397852338804471, 0.001397739925985545, 0.0013976275131666193, 0.0013975151003476933, 0.0013974026875287673, 0.0013972902747098413, 0.0013971778618909153, 0.0013970654490719893, 0.0013969530362530633, 0.0013968406234341373, 0.0013967282106152115, 0.0013966157977962856, 0.0013965033849773596]
  out "initial x":dbl=0.0015088037910843937
  out "Final x":dbl=0.0013965033849773596
  in  "Volts/pixel":dbl=-0.0002
  out "Xin":dbl=0.0015088037910843937
  out "Yin":dbl=-0.007933120791494438
  in  "Correction":dbl[][](array[numeric])=[[500.0, 550.0, 8.0, -1.0], [550.0, 590.0, 20.0, -4.0]]
  in  "Scan mirrors out":tag="Dev1/ao1:0"
  in  "Scan Mirrors in":tag="Dev1/ai1:2"
  in  "Voltage B":dbl min=-10.0 max=10.0 step=0.1 format="%0.2f"
  in  "Voltage A":dbl min=-10.0 max=10.0 step=0.1 format="%0.2f"
  in  "Output B":tag="Dev1/ao3"
  in  "Output A":tag="Dev1/ao2"
  in  "Input Channel":tag="Dev1/ai6"
  in  "Current":bool
  in  "Power":bool=TRUE
  out "ScanGraph":cluster{dbl[], dbl[]}(graph)={[499.989, 504.988, 509.986, 514.984, 519.999, 524.996, 529.993, 534.99, 539.986, 544.998, 549.994, 554.99, 559.984, 564.995, 569.99, 574.983, 579.993, 584.986, 589.994, 594.986, 599.995, 604.986, 609.993, 614.983, 619.99, 624.995, 629.985, 634.99, 639.994], [4.865306176e-06, 4.426406141e-06, 2.1976425389999998e-06, 3.62626727785e-06, 4.471631584e-06, -1.4674275871e-06, 2.5364671989e-06, 3.2164805046e-06, -4.786285424e-06, 4.546786033e-06, -2.0231638244e-06, 3.0966043978e-06, 5.4053851169e-06, 1.89029350225e-06, -8.325836860000001e-07, 5.628519417e-07, 1.2469052133e-06, -1.4945361278600003e-06, 2.74686667808e-06, 3.7131121660000015e-07, 2.0647405537e-06, 1.7817209099999997e-07, 2.10948271503e-06, 1.0479730683000001e-06, 2.8708853302e-06, 1.8259718868e-06, 2.10715707039e-06, 8.843115453999999e-07, 1.9754551140000005e-07]}
  in  "Sensitivity":dbl=1e-09 caption="(A/V)" format="%#_6p"
  out "Readout":dbl=-1.06034975e-06 format="%^#_9e"
  in  "Scan Save Path":path
  in  "On":bool=TRUE
  out "Waveform Chart":dbl(graph)=-1.06034975e-06
  in  "Save":bool
  in  "Exit":bool
  in  "STOP":bool
  in  "Step Time (sec)":dbl=1.0 min=0.001 max=300.0 step=0.001 format="%.3f"
  in  "Step Size (nm)":dbl=5.0 min=0.1 max=100.0 step=0.1 format="%.1f"
  in  "End":dbl=2000.0 min=0.0 max=2000.0 step=0.1 format="%.1f"
  in  "Start":dbl=500.0 min=0.0 max=2000.0 step=0.1 format="%.1f"
  in  "Scan":bool
  in  "Up":bool=TRUE caption="Down"
  in  "Increment (nm)":dbl=10.0 min=0.1 max=2000.0 step=0.1 format="%.1f"
  in  "PMD Settings":T1={"Beam Diameter (mm)"=4.0, "BWIn"=0, "Averaging Rate"=300, "Auto Range"=TRUE} {"Averaging Rate" min=33 max=5000 step=1; "BWIn" items=["HIGH", "LOW"]; "Beam Diameter (mm)" min=1.0 max=9.0 step=0.5}
  in  "Step":bool
  out "Busy":bool
  in  "Send Command":bool
  in  "Command":u16(ring)=1 items=["nm", "goto", "nm/min", "VIS grating", "IR grating"]
  in  "Wavelength (nm)":dbl=640.0 min=0.0 max=2000.0 step=0.1 format="%.1f"
  in  "Scan Speed (nm/min)":dbl=100.0 min=1.0 max=500.0 step=0.1 format="%.1f"
  out "Done?":string="  ok\r\n"
  in  "Send Question":bool
  in  "Ask?":u16(ring) items=["?nm", "?nm/min", "?grating", "?turret", "?gratings"]
  in  "Zero?":bool
  out "PM Error log":string
  out "AUTO?":bool
  out "Zero Value":dbl format="%#.3p"
  out "Rng":string
  in  "Range":i16=1 min=1 max=6 step=1
  in  "Mono Port":refnum<visa-resource-name>="COM11"
  out "IDN String":string="Thorlabs,PM100USB,P2000362,1.3.0\n"
  out "Sensor SN":string="10061433"
  out "Sensor Name":string="S120C"
  out "Reply":string=" 639.994 nm  ok\r\n" caption="Mono Response"
  # "Range Settings"
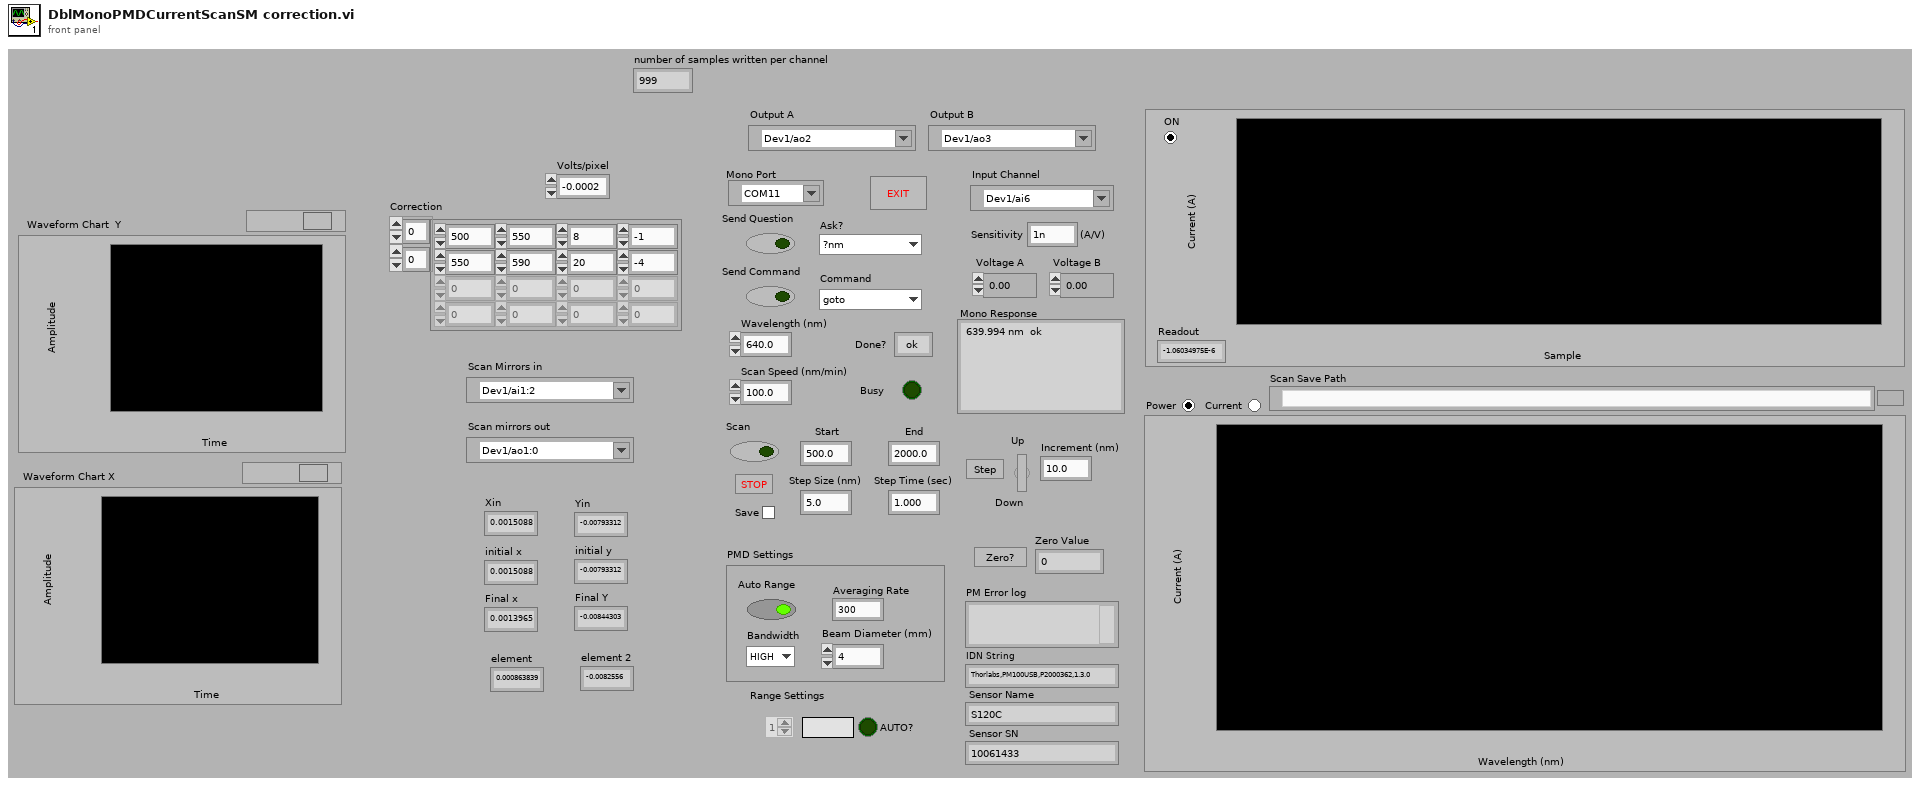
[diagram p1: front panel]
types:
  T1 = cluster{"Beam Diameter (mm)":dbl, "BWIn":u16, "Averaging Rate":i32, "Auto Range":bool}
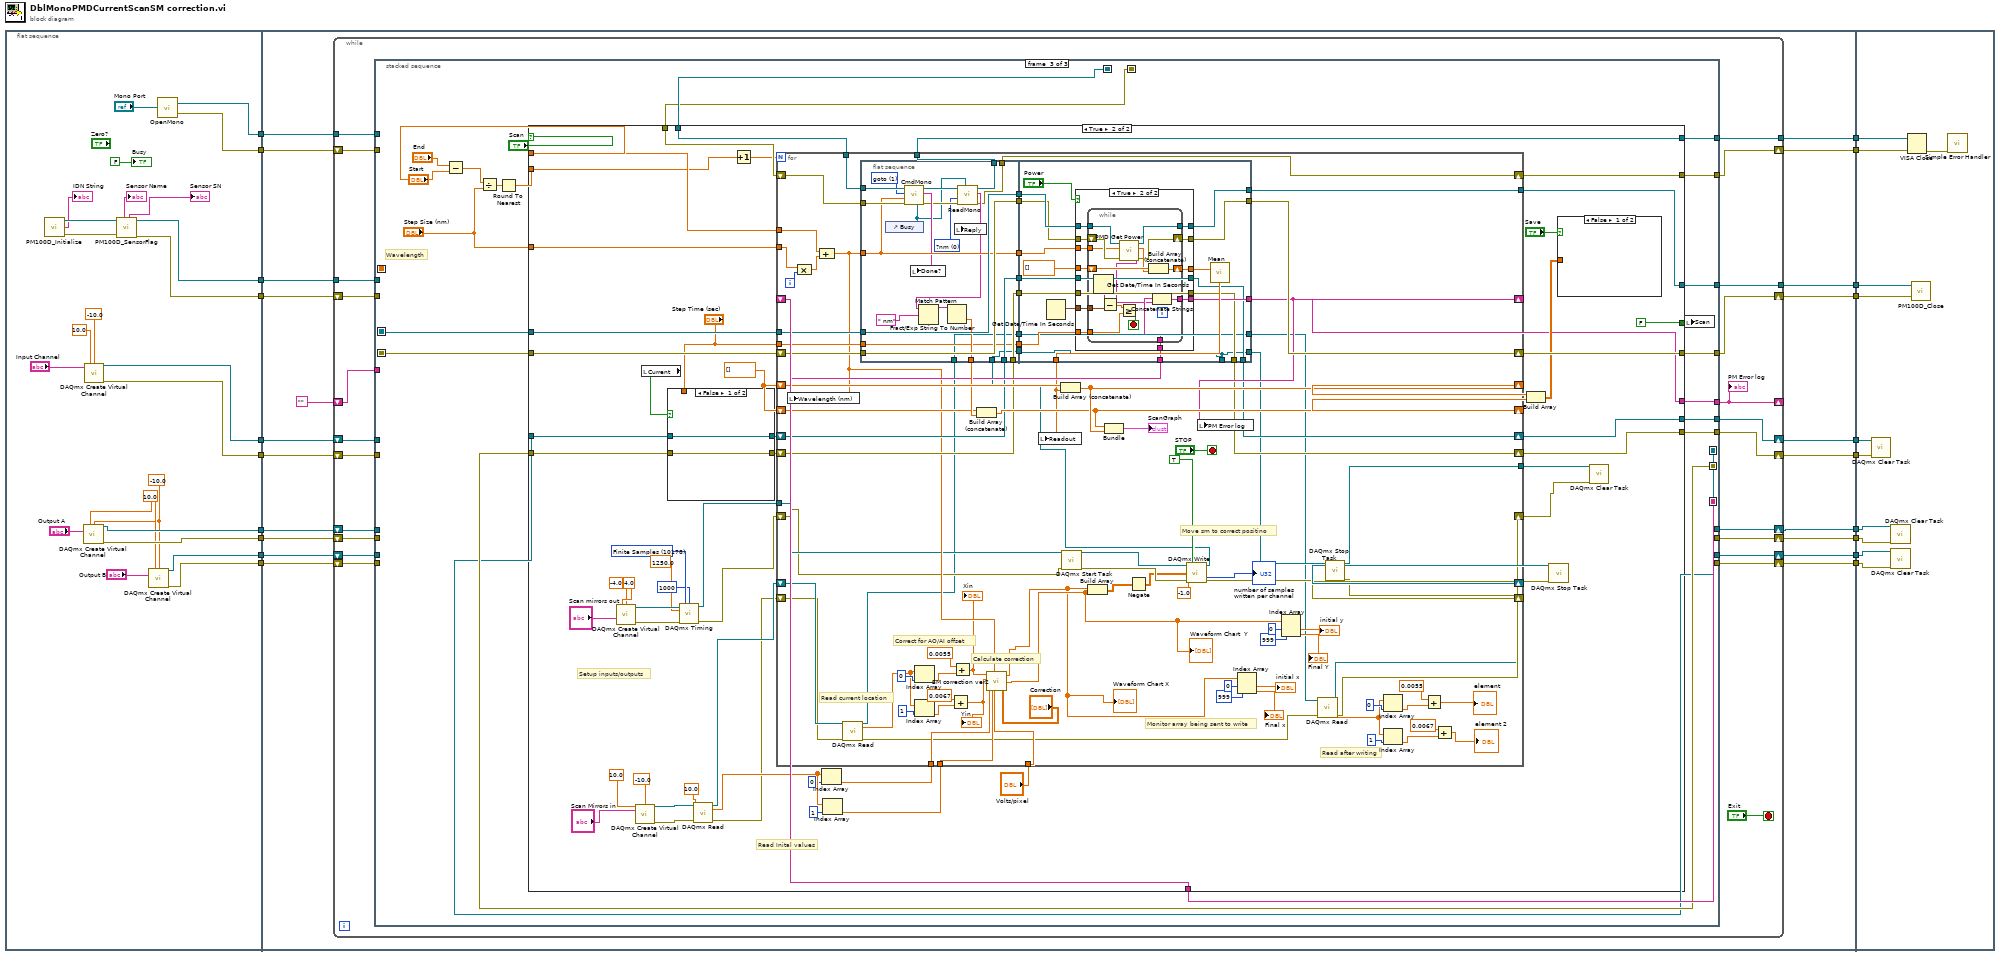
[diagram p0: block diagram]
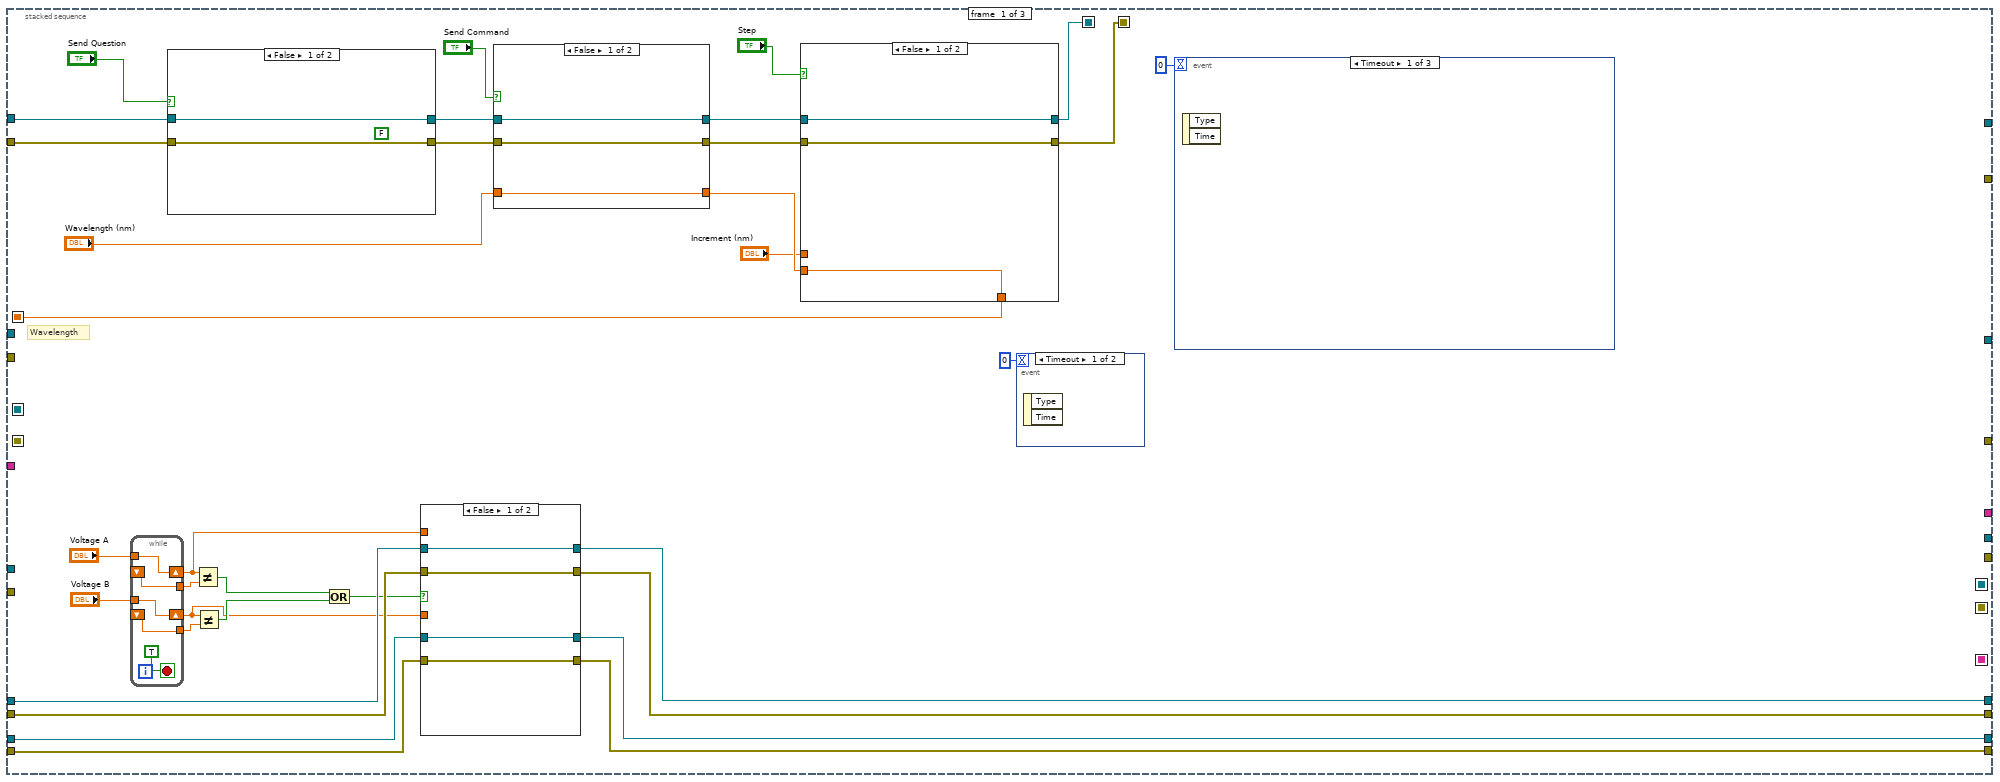
[diagram p2: hidden frame]
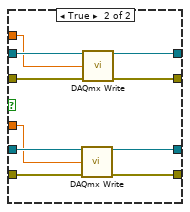
[diagram p3: hidden frame]
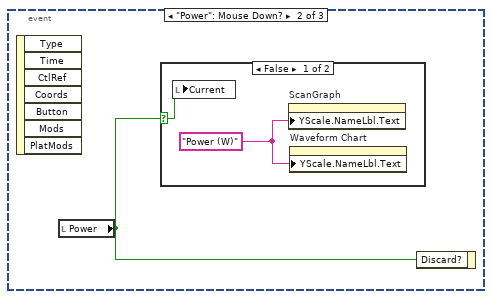
[diagram p4: hidden frame]
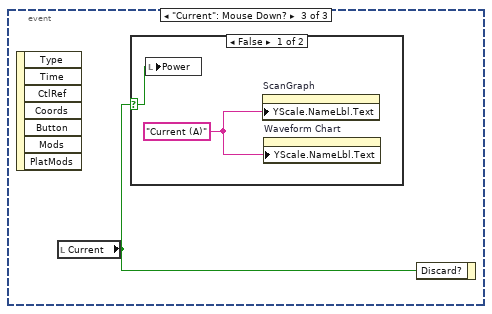
[diagram p6: hidden frame]
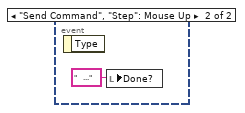
[diagram p8: hidden frame]
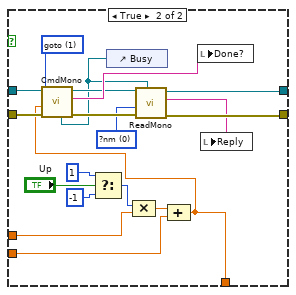
[diagram p9: hidden frame]
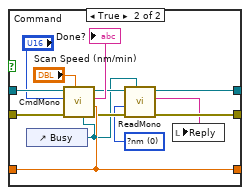
[diagram p10: hidden frame]
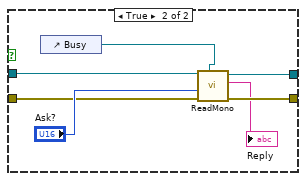
[diagram p11: hidden frame]
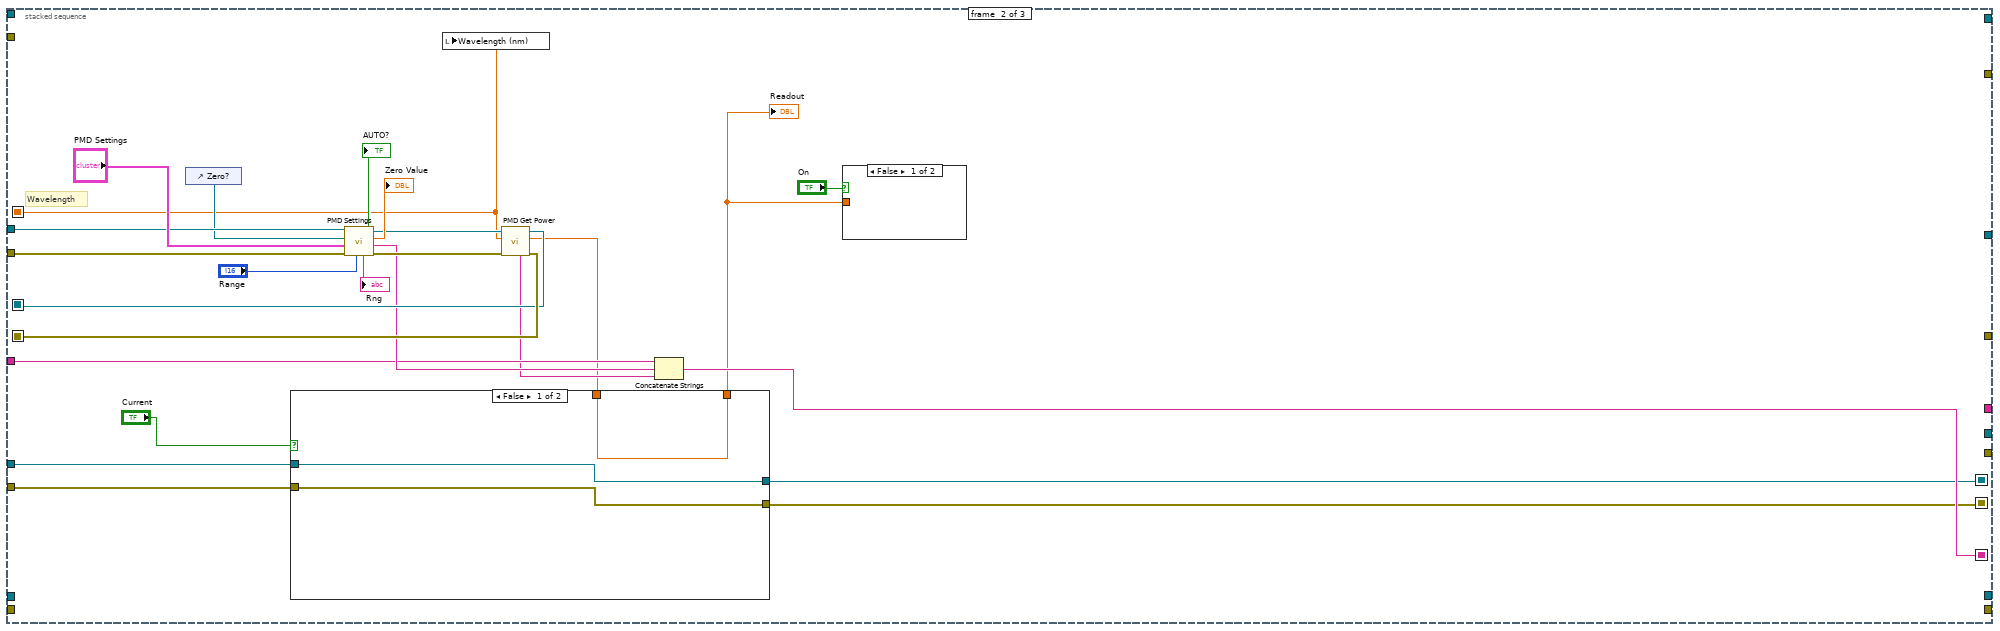
[diagram p12: hidden frame]
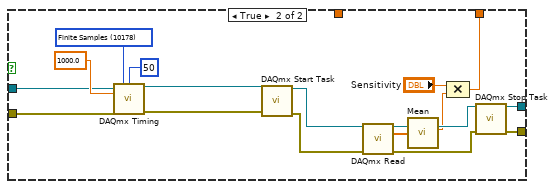
[diagram p13: hidden frame]
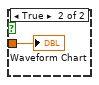
[diagram p14: hidden frame]
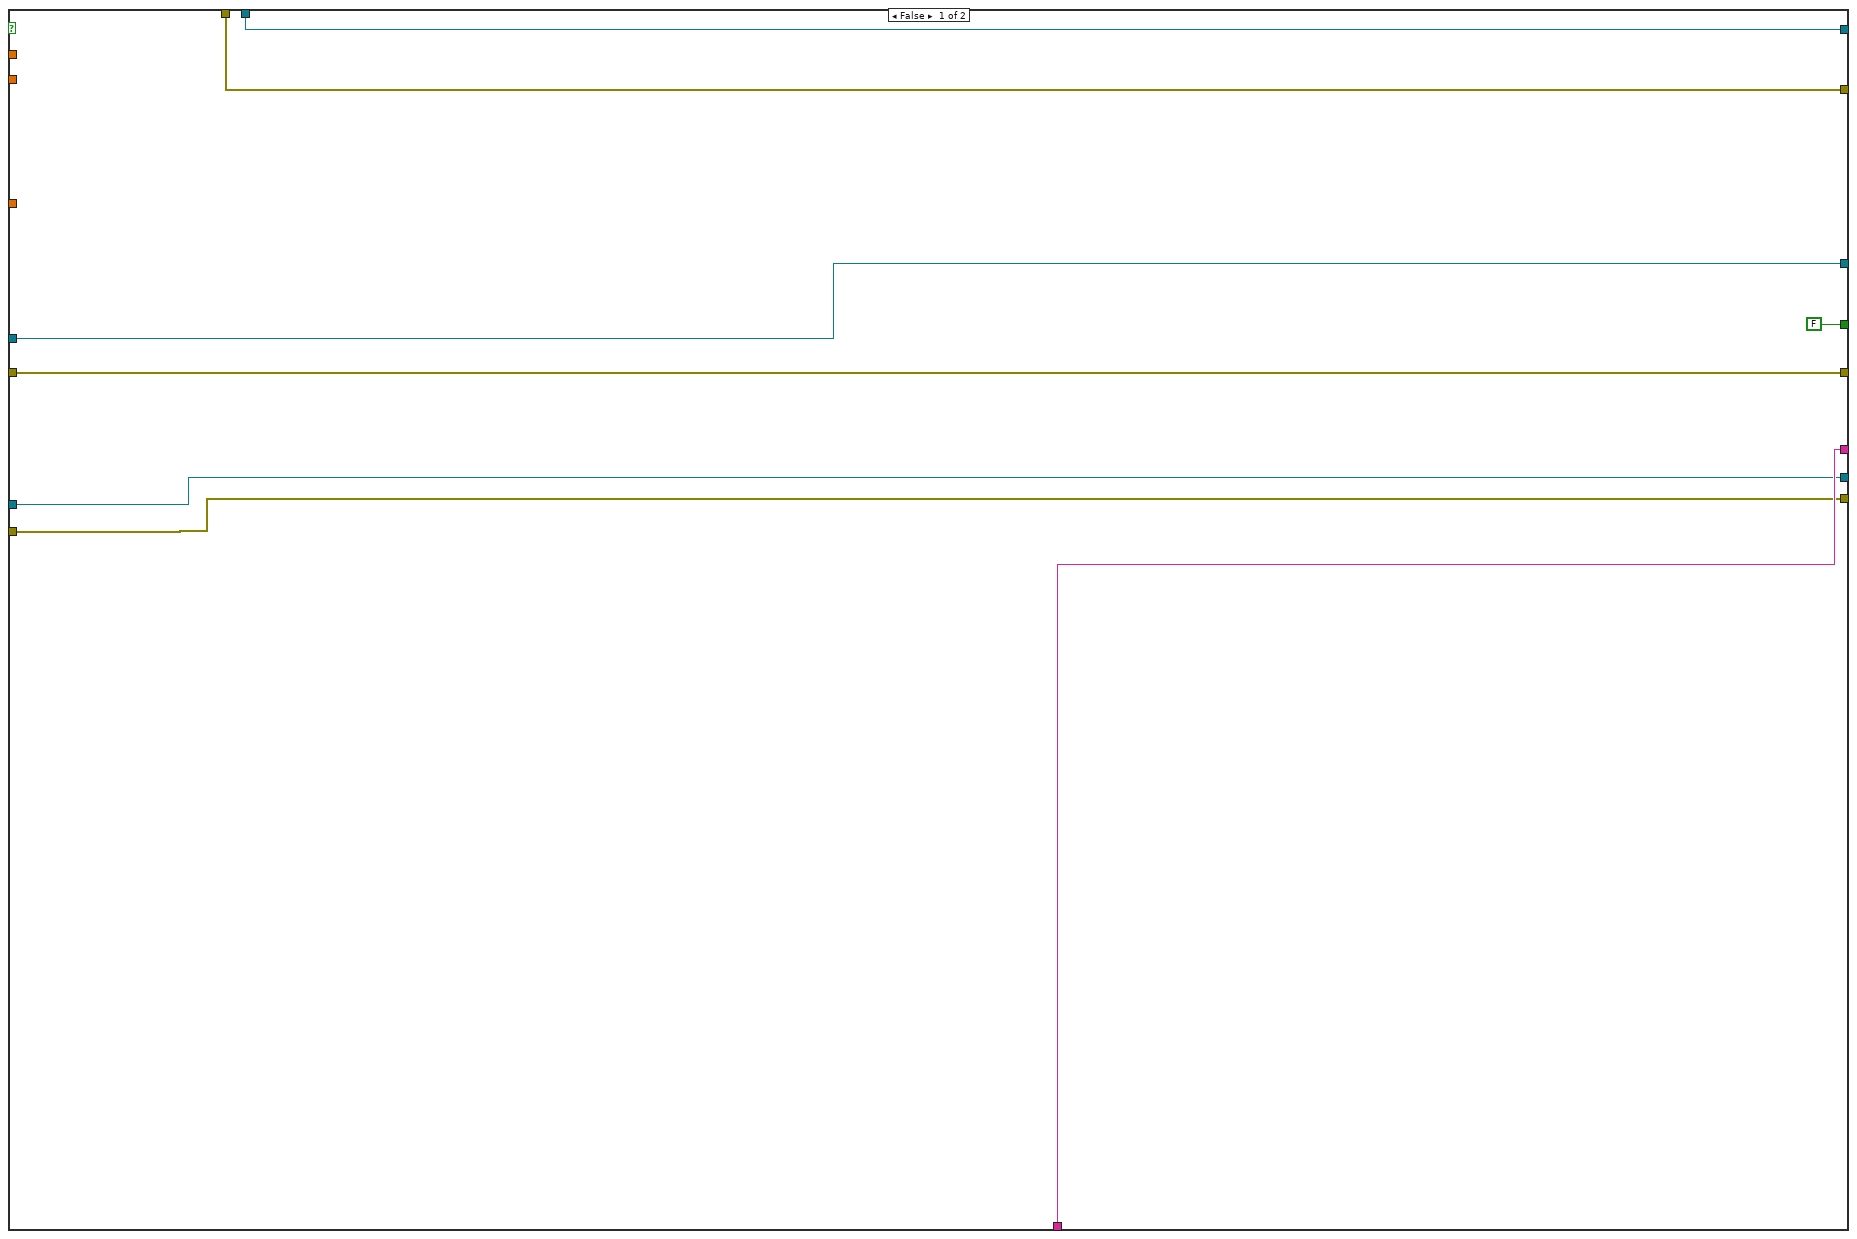
[diagram p15: hidden frame]
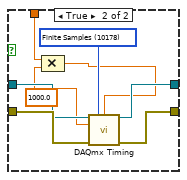
[diagram p16: hidden frame]
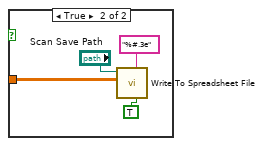
[diagram p17: hidden frame]
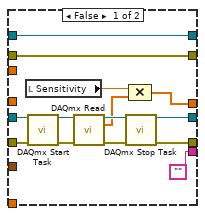
[diagram p18: hidden frame]
diagram:
  n1 = flat-sequence {
    tunnel: [w39] -> w20
    tunnel: [w38] -> w19
    tunnel: [w37] -> w18
    tunnel: [w36] -> w17
    tunnel: [w23] -> w12
    tunnel: [w24] -> w9
    tunnel: [w29] -> w8
    tunnel: [w30] -> w7
    tunnel: [w28] -> w6
    tunnel: [w27] -> w5
    tunnel: w20 -> [w64]
    tunnel: w19 -> [w65]
    tunnel: w18 -> [w63]
    tunnel: w17 -> [w62]
    tunnel: [w61] -> w16
    tunnel: [w60] -> w15
    tunnel: [w59] -> w14
    tunnel: [w58] -> w13
    tunnel: w12 -> [w55]
    tunnel: [w46] -> w11
    tunnel: [w45] -> w10
    tunnel: w9 -> [w56]
    tunnel: w8 -> [w54]
    tunnel: w7 -> [w53]
    tunnel: w6 -> [w52]
    tunnel: w5 -> [w51]
    tunnel: [w47] -> w4
    tunnel: [w48] -> w3
    tunnel: [w49] -> w2
    tunnel: [w50] -> w1
    tunnel: w16 -> [w524]
    tunnel: w15 -> [w523]
    tunnel: w14 -> [w522]
    tunnel: w13 -> [w521]
    tunnel: w11 -> [w519]
    tunnel: w10 -> [w520]
    tunnel: w4 -> [w518]
    tunnel: w3 -> [w517]
    tunnel: w2 -> [w516]
    tunnel: w1 -> [w515]
    frame #0 {
      w25 = -10.0 ("minimum value")
      w26 = 10.0 ("maximum value")
      n2 = call "PM100D_Initialize.vi"() -> ("error out"=w43:errorcluster, "Instrument"=→"IDN String":string, "VISA out"=w44:refnum<visa-resource-name>)  [unwired: 2 in, 1 out]
      n3 = call-poly <vilib>:"DAQmx Create Virtual Channel.vi"("maximum value"=w26, "minimum value"=w25, "physical channels"="Output A") -> ("task out"=w30:refnum<k21>, "error out"=w29:errorcluster)  [unwired: 11 in]
      n4 = call-poly <vilib>:"DAQmx Create Virtual Channel.vi"("maximum value"=10.0, "minimum value"=-10.0, "physical channels"="Input Channel") -> ("task out"=w24:refnum<k21>, "error out"=w23:errorcluster)  [unwired: 11 in]
      n5 = call "PM100D_SensorFlag.vi"("error in (no error)"=w43, "VISA in"=w44) -> ("error out"=w39:errorcluster, "VISA out"=w38:refnum<visa-resource-name>, "sn"=→"Sensor SN":string, "name"=→"Sensor Name":string)  [unwired: 2 in, 4 out]
      n6 = call-poly <vilib>:"DAQmx Create Virtual Channel.vi"("maximum value"=w26, "minimum value"=w25, "physical channels"="Output B") -> ("task out"=w27:refnum<k21>, "error out"=w28:errorcluster)  [unwired: 11 in]
      n7 = call "OpenMono.vi"("Mono Port"="Mono Port") -> ("VISA resource name out"=w37:refnum<visa-resource-name>, "error out"=w36:errorcluster)
      "Busy" <- FALSE ("Busy")
    }
    frame #1 {
      n8 = while {
        tunnel: w65 -> [w86]
        tunnel: w63 -> [w88]
        tunnel: [w83] -> w60
        tunnel: [w81] -> w58
        shift-right: [w80] -> w59
        shift-left: w64 -> [w85]
        shift-right: [w82] -> w61
        shift-left: w62 -> [w87]
        shift-right: [w78] -> _
        shift-left: "" -> [w79]
        shift-right: [w67] -> w45
        shift-left: w55 -> [w76]
        shift-right: [w66] -> w46
        shift-left: w56 -> [w77]
        shift-right: [w68] -> w50
        shift-left: w53 -> [w75]
        shift-right: [w69] -> w49
        shift-left: w54 -> [w74]
        shift-right: [w70] -> w48
        shift-left: w51 -> [w72]
        shift-right: [w71] -> w47
        shift-left: w52 -> [w73]
        stop <- "Exit" stop-if-true
        n9 = stacked-sequence {
          seq-local: [w107 _ _] -> [_ w203 _]
          seq-local: [w112 _ _] -> [_ _ w256]
          seq-local: [w111 _ _] -> [_ _ w255]
          seq-local: [_ w210 _] -> [_ _ w254]
          seq-local: [_ w211 _] -> [_ _ w253]
          seq-local: [_ w204 _] -> [_ _ w247]
          seq-local: [_ w198 _] -> [_ _ w243]
          seq-local: [_ w199 _] -> [_ _ w242]
          tunnel: w88 -> [w118 _ _]
          tunnel: w87 -> [w117 _ _]
          tunnel: w86 -> [_ w213 _]
          tunnel: w85 -> [_ w212 _]
          tunnel: [_ _ w252] -> w83
          tunnel: [_ _ w251] -> w82
          tunnel: [_ _ w250] -> w81
          tunnel: [_ _ w249] -> w80
          tunnel: w79 -> [_ w206 _]
          tunnel: [_ _ w246] -> w78
          tunnel: w77 -> [_ w197 _]
          tunnel: w76 -> [_ w196 _]
          tunnel: [_ _ w245] -> w66
          tunnel: [_ _ w244] -> w67
          tunnel: w75 -> [w102 _ _]
          tunnel: w74 -> [w103 _ _]
          tunnel: w73 -> [w105 _ _]
          tunnel: w72 -> [w104 _ _]
          tunnel: [w101 _ _] -> w71
          tunnel: [w100 _ _] -> w70
          tunnel: [w99 _ _] -> w69
          tunnel: [w98 _ _] -> w68
          frame #0 {
            # "Wavelength"
            n10 = while {
              shift-right: [w140] -> w89
              shift-left: _ -> [w139]
              tunnel: "Voltage B" -> [w140]
              tunnel: [w139] -> w94
              tunnel: "Voltage A" -> [w138]
              shift-right: [w138] -> w90
              shift-left: _ -> [w137]
              tunnel: [w137] -> w95
              stop <- TRUE stop-if-true
            }
            n11 = case shown="False" "Send Question" {
              tunnel: w118 -> [w188 w194]
              tunnel: w117 -> [w187 w193]
              tunnel: [w188 w192] -> w120
              tunnel: [w187 w191] -> w119
              frame False {
                (unwired) FALSE ("Read Error")
              }
              frame True {
                n12 = control-ref of="Busy"() -> (w189:refnum<vi>)
                n13 = call "ReadMono.vi"("Busy"=w189, "error in (no error)"=w193, "Cmd"="Ask?", "Mono Port"=w194) -> ("error out"=w191:errorcluster, "Response"=→"Reply":string, "Mono Port Out"=w192:refnum<visa-resource-name>)  [unwired: 2 in, 1 out]
              }
            }
            n14 = Not Equal?(x=w90, y=w95) -> (x != y?=w93:bool)
            n15 = Not Equal?(x=w89, y=w94) -> (x != y?=w92:bool)
            n16 = Or(x=w93, y=w92) -> (x .or. y?=w91:bool)
            n17 = case shown="False" w91 {
              tunnel: w105 -> [w123 w136]
              tunnel: w104 -> [w124 w135]
              tunnel: w103 -> [w125 w134]
              tunnel: w102 -> [w126 w133]
              tunnel: [w123 w132] -> w101
              tunnel: [w124 w131] -> w100
              tunnel: [w125 w130] -> w99
              tunnel: [w126 w129] -> w98
              tunnel: w90 -> [_ w127]
              tunnel: w89 -> [_ w128]
              frame False {
              }
              frame True {
                n18 = call-poly <vilib>:"DAQmx Write.vi"("task/channels in"=w135, "data"=w128, "error in"=w136) -> ("task out"=w131:refnum<k21>, "error out"=w132:errorcluster)  [unwired: 10 in, 1 out]
                n19 = call-poly <vilib>:"DAQmx Write.vi"("task/channels in"=w133, "data"=w127, "error in"=w134) -> ("task out"=w129:refnum<k21>, "error out"=w130:errorcluster)  [unwired: 10 in, 1 out]
              }
            }
            n20 = case shown="False" "Send Command" {
              tunnel: w120 -> [w173 w186]
              tunnel: w119 -> [w172 w185]
              tunnel: [w173 w178] -> w115
              tunnel: [w172 w177] -> w114
              tunnel: "Wavelength (nm)" -> [w171 w181]
              tunnel: [w171 w181] -> w113
              frame False {
              }
              frame True {
                w176 = u16 0 items=["?nm", "?nm/min", "?grating", "?turret", "?gratings"] ("Cmd")
                n21 = control-ref of="Busy"() -> (w174:refnum<vi>)
                n22 = call "CmdMono.vi"("Busy"=w174, "Scan Speed (nm/min)"="Scan Speed (nm/min)", "error in (no error)"=w185, "Wavelength (nm)"=w181, "Cmd"="Command", "Mono Port"=w186) -> ("error out"=w179:errorcluster, "Response"=→"Done?":string, "Mono Port Out"=w180:refnum<visa-resource-name>)  [unwired: 2 in, 1 out]
                n23 = call "ReadMono.vi"("Busy"=w174, "error in (no error)"=w179, "Cmd"=w176, "Mono Port"=w180) -> ("error out"=w177:errorcluster, "Response"=w175:string, "Mono Port Out"=w178:refnum<visa-resource-name>)  [unwired: 2 in, 1 out]
                n24 = local write "Reply"(w175) -> ()
              }
            }
            n25 = case shown="False" "Step" {
              tunnel: w115 -> [w151 w170]
              tunnel: w114 -> [w150 w169]
              tunnel: w113 -> [w149 w163]
              tunnel: [w151 w156] -> w112
              tunnel: [w150 w157] -> w111
              tunnel: "Increment (nm)" -> [_ w162]
              tunnel: [w149 w152] -> w107
              frame False {
              }
              frame True {
                w154 = u16 0 items=["?nm", "?nm/min", "?grating", "?turret", "?gratings"] ("Cmd")
                w161 = u16 1 items=["nm", "goto", "nm/min", "VIS grating", "IR grating"] ("Cmd")
                n26 = Select(t=1, s="Up", f=-1) -> (s? t:f=w168:i32)
                n27 = control-ref of="Busy"() -> (w153:refnum<vi>)
                n28 = Compound Arithmetic op=MULTIPLY(w168, w162) -> (w164:dbl)
                n29 = Compound Arithmetic op=ADD(w164, w163) -> (w152:dbl)
                n30 = call "CmdMono.vi"("Busy"=w153, "error in (no error)"=w169, "Wavelength (nm)"=w152, "Cmd"=w161, "Mono Port"=w170) -> ("error out"=w158:errorcluster, "Response"=w160:string, "Mono Port Out"=w159:refnum<visa-resource-name>)  [unwired: 3 in, 1 out]
                n31 = call "ReadMono.vi"("Busy"=w153, "error in (no error)"=w158, "Cmd"=w154, "Mono Port"=w159) -> ("error out"=w157:errorcluster, "Response"=w155:string, "Mono Port Out"=w156:refnum<visa-resource-name>)  [unwired: 2 in, 1 out]
                n32 = local write "Done?"(w160) -> ()
                n33 = local write "Reply"(w155) -> ()
              }
            }
            n34 = event shown="[0] Timeout" {
              selector: _ -> [_ _]
              dyn-events: _ -> [_ _]
              timeout: 0 -> [_ _]
              event Timeout {
                n35 = event-data() -> ()  [unwired: 1 in, 2 out]
              }
              event "Send Command", "Step": Mouse Up {
                n36 = event-data() -> ()  [unwired: 1 in, 1 out]
                n37 = local write "Done?"("   ..." ("Done?")) -> ()
              }
            }
            n38 = event shown="[0] Timeout" {
              selector: _ -> [_ _ _]
              dyn-events: _ -> [_ _ _]
              timeout: 0 -> [_ _ _]
              event Timeout {
                n39 = event-data() -> ()  [unwired: 1 in, 2 out]
              }
              event "Power": Mouse Down? {
                n40 = event-data() -> ()  [unwired: 1 in, 7 out]
                n41 = local read "Power"() -> (w142:bool)
                n42 = case shown="False" w142 {
                  selector: w142 -> [w144 _]
                  frame False {
                    w143 = "Power (W)" ("Y Scale.Name Label.Text")
                    n43 = local write "Current"(w144) -> ()
                    n44 = property on="ScanGraph" class="XYGraph (strict)"("YScale.NameLbl.Text"=w143) -> ()  [unwired: 2 in, 2 out]
                    n45 = property on="Waveform Chart" class="WFChart (strict)"("YScale.NameLbl.Text"=w143) -> ()  [unwired: 2 in, 2 out]
                  }
                  frame True {
                  }
                }
                n46 = event-data("Discard?"=w142) -> ()  [unwired: 1 in, 1 out]
              }
              event "Current": Mouse Down? {
                n47 = event-data() -> ()  [unwired: 1 in, 7 out]
                n48 = local read "Current"() -> (w145:bool)
                n49 = case shown="False" w145 {
                  selector: w145 -> [w146 _]
                  frame False {
                    w147 = "Current (A)" ("Y Scale.Name Label.Text")
                    n50 = local write "Power"(w146) -> ()
                    n51 = property on="ScanGraph" class="XYGraph (strict)"("YScale.NameLbl.Text"=w147) -> ()  [unwired: 2 in, 2 out]
                    n52 = property on="Waveform Chart" class="WFChart (strict)"("YScale.NameLbl.Text"=w147) -> ()  [unwired: 2 in, 2 out]
                  }
                  frame True {
                  }
                }
                n53 = event-data("Discard?"=w145) -> ()  [unwired: 1 in, 1 out]
              }
            }
          }
          frame #1 {
            # "Wavelength"
            n54 = control-ref of="Zero?"() -> (w208:refnum<vi>)
            n55 = call "PMD Settings.vi"("Visa In"=w213, "Zero?"=w208, "PMD Settings In"="PMD Settings", "Error In"=w212, "Range"="Range") -> ("AUTO?"=→"AUTO?":bool, "Rng"=→"Rng":string, "Visa Out"=w216:refnum<visa-resource-name>, "ZeroValue"=→"Zero Value":dbl, "PM Error log"=w207:string, "error out"=w215:errorcluster)
            n56 = local write "Wavelength (nm)"(w203) -> ()
            n57 = call "PMD Get Power.vi"("VISA In"=w216, "Wavelength (nm)"=w203, "error in"=w215) -> ("PMD Error"=w205:string, "VISA out"=w210:refnum<visa-resource-name>, "Readout value"=w202:dbl, "error out"=w211:errorcluster)  [unwired: 1 in, 2 out]
            n58 = case shown="False" "Current" {
              tunnel: w202 -> [w223 _]
              tunnel: w197 -> [w222 w226]
              tunnel: w196 -> [w221 w227]
              tunnel: [w223 w239] -> w200
              tunnel: [w221 w235] -> w198
              tunnel: [w222 w236] -> w199
              frame False {
              }
              frame True {
                w229 = 10178 items=["Finite Samples"=10178, "Continuous Samples"=10123, "Hardware Timed Single Point"=12522] ("sample mode")
                n59 = call-poly <vilib>:"DAQmx Timing.vi"("task/channels in"=w226, "sample mode"=w229, "samples per channel"=50, "rate"=1000.0, "error in"=w227) -> ("task out"=w225:refnum<k21>, "error out"=w224:errorcluster)  [unwired: 9 in]
                n60 = call <vilib>:"DAQmx Start Task.vi"("task/channels in"=w225, "error in"=w224) -> ("task out"=w237:refnum<k21>, "error out"=w238:errorcluster)  [unwired: 12 in]
                n61 = call-poly <vilib>:"DAQmx Read.vi"("task/channels in"=w237, "error in"=w238) -> ("task out"=w233:refnum<k21>, "data"=w232:dbl[], "error out"=w234:errorcluster)  [unwired: 11 in]
                n62 = call <vilib>:"Mean.vi"("X"=w232) -> ("mean"=w231:dbl)  [unwired: 1 out]
                n63 = Compound Arithmetic op=MULTIPLY("Sensitivity", w231) -> (w239:dbl)
                n64 = call <vilib>:"DAQmx Stop Task.vi"("task/channels in"=w233, "error in"=w234) -> ("task out"=w236:refnum<k21>, "error out"=w235:errorcluster)  [unwired: 12 in]
              }
            }
            "Readout" <- w200
            n65 = Concatenate Strings(w206, w207, w205) -> (w204:string)
            n66 = case shown="False" "On" {
              tunnel: w200 -> [_ w241]
              frame False {
              }
              frame True {
                "Waveform Chart" <- w241
              }
            }
          }
          frame #2 {
            # "Wavelength"
            n67 = Subtract(x="End", y="Start") -> (x-y=w261:dbl)
            n68 = Divide(x=w261, y="Step Size (nm)") -> (x/y=w260:dbl)
            n69 = Round To Nearest(number=w260) -> (nearest integer value=w259:dbl)
            n70 = case shown="True" "Scan" {
              tunnel: w259 -> [_ w322]
              tunnel: w255 -> [w269 w324]
              tunnel: w256 -> [w268 w325]
              tunnel: "Start" -> [_ w327]
              tunnel: "Step Size (nm)" -> [_ w326]
              tunnel: w254 -> [w271 w320]
              tunnel: w253 -> [w270 w319]
              tunnel: [w271 w308] -> w250
              tunnel: [w270 w318] -> w249
              tunnel: [w269 w317] -> w251
              tunnel: [w268 w316] -> w252
              tunnel: [FALSE ("Scan") FALSE ("Scan")] -> w248
              tunnel: w247 -> [w266 w310]
              tunnel: [w266 w309] -> w246
              tunnel: [w265 w307] -> w245
              tunnel: [w264 w306] -> w244
              tunnel: w243 -> [w264 w304]
              tunnel: w242 -> [w265 w303]
              frame False {
              }
              frame True {
                w277 = 10178 items=["Finite Samples"=10178, "Continuous Samples"=10123, "Hardware Timed Single Point"=12522] ("sample mode")
                w323 = dbl[] []
                # "Read Inital values"
                # "Setup inputs/outputs"
                n71 = call-poly <vilib>:"DAQmx Create Virtual Channel.vi"("maximum value"=4.0, "minimum value"=-4.0, "physical channels"="Scan mirrors out") -> ("task out"=w285:refnum<k21>, "error out"=w284:errorcluster)  [unwired: 11 in]
                n72 = call-poly <vilib>:"DAQmx Create Virtual Channel.vi"("maximum value"=10.0, "minimum value"=-10.0, "physical channels"="Scan Mirrors in") -> ("task out"=w294:refnum<k21>, "error out"=w298:errorcluster)  [unwired: 11 in]
                n73 = local read "Current"() -> (w305:bool)
                n74 = case shown="False" w305 {
                  tunnel: w304 -> [w328 w336]
                  tunnel: w303 -> [w329 w335]
                  tunnel: [w329 w334] -> w302
                  tunnel: [w328 w333] -> w301
                  tunnel: "Step Time (sec)" -> [_ w332]
                  frame False {
                  }
                  frame True {
                    w337 = 10178 items=["Finite Samples"=10178, "Continuous Samples"=10123, "Hardware Timed Single Point"=12522] ("sample mode")
                    w331 = 1000.0 ("rate")
                    n75 = Compound Arithmetic op=MULTIPLY(w332, w331) -> (w330:dbl)
                    n76 = call-poly <vilib>:"DAQmx Timing.vi"("task/channels in"=w335, "sample mode"=w337, "samples per channel"=w330, "rate"=w331, "error in"=w336) -> ("task out"=w334:refnum<k21>, "error out"=w333:errorcluster)  [unwired: 9 in]
                  }
                }
                n77 = call-poly <vilib>:"DAQmx Timing.vi"("task/channels in"=w285, "sample mode"=w277, "samples per channel"=1000, "rate"=1250.0, "error in"=w284) -> ("task out"=w274:refnum<k21>, "error out"=w275:errorcluster)  [unwired: 9 in]
                n78 = call-poly <vilib>:"DAQmx Read.vi"("task/channels in"=w294, "timeout"=10.0, "error in"=w298) -> ("task out"=w283:refnum<k21>, "data"=w293:dbl[], "error out"=w282:errorcluster)  [unwired: 10 in]
                n79 = Increment(x=w322) -> (x+1=w321:dbl)
                n80 = Index Array(array=w293, index=0) -> (element=w290:dbl)
                n81 = Index Array(array=w293, index=1) -> (element=w289:dbl)
                n82 = for {
                  N: w321 -> [_]
                  tunnel: w325 -> [w428]
                  tunnel: w327 -> [w424]
                  tunnel: w326 -> [w426]
                  shift-right: [w412] -> w315
                  shift-left: w323 -> [w430]
                  shift-right: [w423] -> w317
                  shift-left: w324 -> [w429]
                  shift-right: [w409] -> w314
                  shift-left: w323 -> [w410]
                  tunnel: w320 -> [w421]
                  shift-right: [w416] -> w318
                  shift-left: w319 -> [w420]
                  tunnel: [w415] -> w308
                  tunnel: [w414] -> w316
                  shift-right: [w407] -> w309
                  shift-left: w310 -> [w408]
                  shift-right: [w404] -> w306
                  shift-left: w301 -> [w399]
                  shift-right: [w403] -> w307
                  shift-left: w302 -> [w400]
                  tunnel: "Step Time (sec)" -> [w401]
                  tunnel: w290 -> [w392]
                  tunnel: w289 -> [w391]
                  shift-right: [w380] -> w272
                  shift-left: w275 -> [w376]
                  shift-right: [w360] -> w281
                  shift-left: w283 -> [w394]
                  shift-right: [w361] -> w280
                  shift-left: w282 -> [w393]
                  tunnel: "Volts/pixel" -> [w388]
                  tunnel: w274 -> [w378]
                  tunnel: [w379] -> w273
                  i -> [w427]
                  stop <- "STOP" stop-if-true
                  # "Monitor array being sent to write"
                  # "Read after writing"
                  # "Calculate correction"
                  # "Correct for AO/AI offset"
                  # "Read current location"
                  # "Move sm to correct positino"
                  n83 = Compound Arithmetic op=MULTIPLY(w426, w427) -> (w425:dbl)
                  n84 = Compound Arithmetic op=ADD(w424, w425) -> (w390:dbl)
                  n85 = local write "Wavelength (nm)"(w390) -> ()
                  n86 = call-poly <vilib>:"DAQmx Read.vi"("task/channels in"=w394, "error in"=w393) -> ("task out"=w365:refnum<k21>, "data"=w395:dbl[], "error out"=w362:errorcluster)  [unwired: 11 in]
                  n87 = flat-sequence {
                    tunnel: w429 -> [w452]
                    tunnel: w428 -> [w451]
                    tunnel: w390 -> [w447]
                    tunnel: [w436] -> w423
                    tunnel: w421 -> [w449]
                    tunnel: w420 -> [w448]
                    tunnel: [w449] -> w419
                    tunnel: [w448] -> w418
                    tunnel: [w447] -> w417
                    tunnel: [w441] -> w414
                    tunnel: [w437] -> w411
                    tunnel: w399 -> [w434]
                    tunnel: [w435] -> w406
                    tunnel: w400 -> [w435]
                    tunnel: [w434] -> w405
                    tunnel: [w433] -> w402
                    tunnel: w401 -> [w433]
                    tunnel: w368 -> [w432]
                    tunnel: [w432] -> w367
                    tunnel: w365 -> [w431]
                    tunnel: [w431] -> w364
                    tunnel: [w468] -> w398
                    tunnel: w419 -> [w467]
                    tunnel: w418 -> [w466]
                    tunnel: w417 -> [w465]
                    tunnel: [w461] -> w416
                    tunnel: [w464] -> w415
                    tunnel: w408 -> [w463]
                    tunnel: [w462] -> w407
                    tunnel: w406 -> [w459]
                    tunnel: w405 -> [w458]
                    tunnel: [w456] -> w403
                    tunnel: [w457] -> w404
                    tunnel: w402 -> [w460]
                    tunnel: [w454] -> _
                    tunnel: [w454] -> w374
                    tunnel: w367 -> [w454]
                    tunnel: [w453] -> w363
                    tunnel: w364 -> [w453]
                    frame #0 {
                      w443 = u16 0 items=["?nm", "?nm/min", "?grating", "?turret", "?gratings"] ("Cmd")
                      w450 = u16 1 items=["nm", "goto", "nm/min", "VIS grating", "IR grating"] ("Cmd")
                      n88 = control-ref of="Busy"() -> (w442:refnum<vi>)
                      n89 = call "CmdMono.vi"("Busy"=w442, "error in (no error)"=w452, "Wavelength (nm)"=w447, "Cmd"=w450, "Mono Port"=w451) -> ("error out"=w444:errorcluster, "Response"=w446:string, "Mono Port Out"=w445:refnum<visa-resource-name>)  [unwired: 3 in, 1 out]
                      n90 = local write "Done?"(w446) -> ()
                      n91 = call "ReadMono.vi"("Busy"=w442, "error in (no error)"=w444, "Cmd"=w443, "Mono Port"=w445) -> ("error out"=w436:errorcluster, "Response"=w439:string, "Mono Port Out"=w441:refnum<visa-resource-name>)  [unwired: 2 in, 1 out]
                      n92 = Match Pattern(string=w439, regular expression=" nm") -> (before substring=w438:string)  [unwired: 1 in, 3 out]
                      n93 = Fract/Exp String To Number(string=w438) -> (number=w437:dbl)  [unwired: 3 in, 1 out]
                      n94 = local write "Reply"(w439) -> ()
                    }
                    frame #1 {
                      n95 = Get Date/Time In Seconds() -> (seconds since 1Jan1904=w470:timestamp)
                      n96 = case shown="True" "Power" {
                        tunnel: dbl[] [] -> [_ w498]
                        tunnel: w470 -> [_ w497]
                        tunnel: [w472 w496] -> w469
                        tunnel: w467 -> [w484 w495]
                        tunnel: w466 -> [w483 w494]
                        tunnel: w465 -> [_ w493]
                        tunnel: [w484 w492] -> w464
                        tunnel: w463 -> [_ w491]
                        tunnel: ["" w490] -> w462
                        tunnel: [w483 w489] -> w461
                        tunnel: w460 -> [_ w488]
                        tunnel: w459 -> [w482 w486]
                        tunnel: w458 -> [w481 w487]
                        tunnel: [w476 w487] -> w457
                        tunnel: [w475 w486] -> w456
                        frame False {
                          n97 = local read "Sensitivity"() -> (w473:dbl)
                          n98 = call <vilib>:"DAQmx Start Task.vi"("task/channels in"=w482, "error in"=w481) -> ("task out"=w480:refnum<k21>, "error out"=w479:errorcluster)  [unwired: 12 in]
                          n99 = call-poly <vilib>:"DAQmx Read.vi"("task/channels in"=w480, "error in"=w479) -> ("task out"=w478:refnum<k21>, "data"=w474:dbl[], "error out"=w477:errorcluster)  [unwired: 11 in]
                          n100 = call <vilib>:"DAQmx Stop Task.vi"("task/channels in"=w478, "error in"=w477) -> ("task out"=w475:refnum<k21>, "error out"=w476:errorcluster)  [unwired: 12 in]
                          n101 = Compound Arithmetic op=MULTIPLY(w473, w474) -> (w472:dbl[])
                        }
                        frame True {
                          n102 = while {
                            shift-right: [w513] -> w496
                            shift-left: w498 -> [w514]
                            tunnel: w497 -> [w511]
                            tunnel: w495 -> [w506]
                            tunnel: w493 -> [w502]
                            tunnel: [w504] -> w492
                            tunnel: w491 -> [w508]
                            tunnel: [w507] -> w490
                            shift-right: [w500] -> w489
                            shift-left: w494 -> [w505]
                            tunnel: w488 -> [w499]
                            stop <- w509 stop-if-true
                            n103 = Get Date/Time In Seconds() -> (seconds since 1Jan1904=w512:timestamp)
                            n104 = Subtract(x=w512, y=w511) -> (x-y=w510:dbl)
                            n105 = call "PMD Get Power.vi"("VISA In"=w506, "Wavelength (nm)"=w502, "error in"=w505) -> ("PMD Error"=w501:string, "VISA out"=w504:refnum<visa-resource-name>, "Readout value"=w503:dbl, "error out"=w500:errorcluster)  [unwired: 1 in, 2 out]
                            n106 = Greater Or Equal?(x=w510, y=w499) -> (x >= y?=w509:bool)
                            n107 = Build Array (concatenate)(w514, w503) -> (w513:dbl[])
                            n108 = Concatenate Strings(w508, w501) -> (w507:string)
                          }
                        }
                      }
                      n109 = call <vilib>:"Mean.vi"("X"=w469) -> ("mean"=w468:dbl)  [unwired: 1 out]
                    }
                  }
                  n110 = Index Array(array=w395, index=0) -> (element=w353:dbl)
                  n111 = Index Array(array=w395, index=1) -> (element=w350:dbl)
                  n112 = Add(x=0.0067, y=w350) -> (x+y=w348:dbl)
                  "Yin" <- w348
                  n113 = Add(x=0.0055, y=w353) -> (x+y=w351:dbl)
                  "Xin" <- w351
                  n114 = Build Array (concatenate)(w410, w411) -> (w409:dbl[])
                  n115 = call "SM correction ver2.vi"("V in x"=w351, "nm in"=w390, "V in y"=w348, "V x initial"=w392, "Volts/pixel"=w388, "V y initial"=w391, "Array"="Correction") -> ("V out x"=w354:dbl[], "V out y"=w369:dbl[])
                  "Waveform Chart X" <- w354
                  "Waveform Chart  Y" <- w369
                  n116 = local write "Readout"(w398) -> ()
                  n117 = Build Array (concatenate)(w430, w398) -> (w412:dbl[])
                  n118 = call <vilib>:"DAQmx Start Task.vi"("task/channels in"=w378, "error in"=w376) -> ("task out"=w377:refnum<k21>, "error out"=w375:errorcluster)  [unwired: 12 in]
                  n119 = Build Array(w354, w369) -> (w356:dbl[][])
                  n120 = Bundle(w409, w412) -> (→"ScanGraph":cluster{dbl[], dbl[]})  [unwired: 1 in]
                  n121 = Negate(x=w356) -> (-x=w355:dbl[][])
                  n122 = call-poly <vilib>:"DAQmx Write.vi"("task/channels in"=w377, "auto start"=TRUE, "data"=w355, "timeout"=-1.0, "error in"=w375) -> ("task out"=w368:refnum<k21>, "number of samples written per channel"=→"number of samples written per channel":u32, "error out"=w381:errorcluster)  [unwired: 8 in]
                  n123 = local write "PM Error log"(w407) -> ()
                  n124 = Index Array(array=w354, index #1=0 ("index"), index #2=999 ("index")) -> (element #1=→"initial x":dbl, element #2=→"Final x":dbl)
                  n125 = Index Array(array=w369, index #1=0 ("index"), index #2=999 ("index")) -> (element #1=→"initial y":dbl, element #2=→"Final Y":dbl)
                  n126 = call-poly <vilib>:"DAQmx Read.vi"("task/channels in"=w363, "error in"=w362) -> ("task out"=w360:refnum<k21>, "data"=w357:dbl[], "error out"=w361:errorcluster)  [unwired: 11 in]
                  n127 = call <vilib>:"DAQmx Stop Task.vi"("task/channels in"=w374, "error in"=w381) -> ("task out"=w379:refnum<k21>, "error out"=w380:errorcluster)  [unwired: 12 in]
                  n128 = Index Array(array=w357, index=0) -> (element=w344:dbl)
                  n129 = Index Array(array=w357, index=1) -> (element=w345:dbl)
                  n130 = Add(x=0.0055, y=w344) -> (x+y=→"element":dbl)
                  n131 = Add(x=0.0067, y=w345) -> (x+y=→"element 2":dbl)
                }
                n132 = Build Array(w315, w314) -> (w313:dbl[][])
                n133 = call <vilib>:"DAQmx Stop Task.vi"("task/channels in"=w281, "error in"=w280) -> ()  [unwired: 12 in, 2 out]
                n134 = case shown="False" "Save" {
                  tunnel: w313 -> [_ w338]
                  frame False {
                  }
                  frame True {
                    n135 = call-poly <vilib>:"Write To Spreadsheet File.vi"("transpose? (no:F)"=TRUE, "format (%.3f)"="%#.3e", "2D data"=w338, "file path (dialog if empty)"="Scan Save Path") -> ()  [unwired: 4 in, 1 out]
                  }
                }
                n136 = call <vilib>:"DAQmx Clear Task.vi"("task in"=w273, "error in"=w272) -> ()  [unwired: 13 in, 1 out]
              }
            }
            n137 = local write "Scan"(w248) -> ()
          }
        }
        "PM Error log" <- w78
      }
    }
    frame #2 {
      n138 = call <vilib>:"DAQmx Clear Task.vi"("task in"=w519, "error in"=w520) -> ()  [unwired: 13 in, 1 out]
      n139 = call <vilib>:"DAQmx Clear Task.vi"("task in"=w515, "error in"=w516) -> ()  [unwired: 13 in, 1 out]
      n140 = call <vilib>:"DAQmx Clear Task.vi"("task in"=w517, "error in"=w518) -> ()  [unwired: 13 in, 1 out]
      n141 = VISA Close(VISA resource name=w523, error in (no error)=w524) -> (error out=w525:errorcluster)
      n142 = call "PM100D_Close.vi"("error in (no error)"=w522, "VISA resource name"=w521) -> ()  [unwired: 2 in]
      n143 = call <vilib>:"Simple Error Handler.vi"("error in (no error)"=w525) -> ()  [unwired: 1 in, 8 out]
    }
  }
